vi "Lockin_time_data analysis.vi"(0 "File or Folder Path":path=path "G:/.shortcut-targets-by-id/0B8-gGFa6hkR4XzJJMDlqZXVKRk0/ansom/Data/PPMS 3/SA40511C.20250205/01-Rwire_BsweepTsweep", 5 "offset":i32, 7 "length":i32=1, 9 "index":T4={"I+(A)"="X2", "I-(A)"="X5", "V4T+"="X1", "V4T-"="X6", "Top gate "="AO3", "Bottom Gate"="AO4", "Local Gate"="AO6", "B/Time"="Time", "X axis"="Magnet", "Temp"="Temperature"}, 11 "stop":bool, 12 "File Type":T3=enum."TDMS", 13 "decimate files":i32=1) -> (6 "V_N vs B":cluster{dbl[], dbl[]}[](graph), 8 "Gvs B":cluster{dbl[], dbl[]}[](graph), 10 "Gates and B":T1={"Top gate"=-2.38250399563554e-06, "Bottom Gate"=0.0, "Local Gate"=0.0, "B"=3821664573.0419946, "X axis"=2.999917578125}, 14 "Comments":string="Device: \r  Device Name: SA40511C.20250205\r  Computer: PPMS3DAQ\r  User: Ranjani\r  Instrument: PPMS 3\r  Description: |\r    LAO/KTO 3wire Nernst\r\rExperiment: \r  Time: 2025-02-06T01:02:54\r  Description: |\r    T = 100mK to 2K, 100mK step\r    B= 3T to -3T, 30Oe/s 0.18T/min\r    \r    Wire 2\r    I+/- = 2/5  1mV@13Hz\r    V+/- = 1/26\r    Wire 1\r    I2+/- = 3/4 1mV@13Hz\r    Wire 3\r\rSweep: \r- Loop1: [OFF, 0.000000]\r- Loop2: [OFF, 0.000000]\r- Loop3: [OFF, 0.000000]\r- Loop4: [OFF, 0.000000]\r\rWiring: \r- Electrode 1: Lockin 1, V1+\r- Electrode 2: Lockin 2, I+\r- Electrode 3: Lockin 3, I2+\r- Electrode 4: Lockin 4, I2-\r- Electrode 5: Lockin 5, I-\r- Electrode 26: Lockin 6, V1-\r- Electrode 27: Lockin 7, I3+\r- Electrode 28: Lockin 8, I2-\r\rLockin: \r  AO: \r  - AO 1: amp = 0.000 mV, DC = 0.000 mV, f = 13.00 Hz, phi = 0.00°, Sine\r  - AO 2: amp = 1.000 mV, DC = 0.000 mV, f = 13.00 Hz, phi = 0.00°, Sine\r  - AO 3: amp = 1.000 mV, DC = 0.000 mV, f = 13.00 Hz, phi = 0.00°, Sine\r  - AO 4: amp = 0.000 mV, DC = 0.000 mV, f = 13.00 Hz, phi = 0.00°, Sine\r  - AO 5: amp = 0.000 mV, DC = 0.000 mV, f = 13.00 Hz, phi = 0.00°, Sine\r  - AO 6: amp = 0.000 mV, DC = 0.000 mV, f = 13.00 Hz, phi = 0.00°, Sine\r  - AO 7: amp = 0.000 mV, DC = 0.000 mV, f = 13.00 Hz, phi = 0.00°, Sine\r  - AO 8: amp = 1.000 mV, DC = 0.000 mV, f = 13.00 Hz, phi = 0.00°, Sine\r  REF: \r  - Lockin 1: f = 13.00 Hz, phi = 0.00°, TC = 0.03 s, order = 2 \r  - Lockin 2: f = 26.00 Hz, phi = 0.00°, TC = 0.03 s, order = 2 \r  Sampling: \r  - Fs: 13000.000000\r  - N: 1000\r")   [LabVIEW 2020]
uses:
  <userlib>/LevyLab/LV-Data/LV-Data/Typedefs/File Type--enum.ctl
  <userlib>/LevyLab/LV-Data/LV-Data/Typedefs/Dictionary--cluster.ctl
  <userlib>/LevyLab/Graph Utilities/graph_utilities.lvclass/graph_utilities.ctl
  <vilib>/Analysis/2dsp.llb/Decimate (single shot, DBL).vi
  <userlib>/LevyLab/XY Utilities/subVIs/Sort (multiple).vi
  <userlib>/LevyLab/XY Utilities/subVIs/Moving Average (multiple).vi
  <userlib>/LevyLab/XY Utilities/subVIs/Moving Average (single).vi
  <userlib>/LevyLab/XY Utilities/Private/X Units.vi
  <userlib>/LevyLab/XY Utilities/Private/X Array Range to Index.vi
  <userlib>/_OpenG.lib/array/array.llb/Sort Array__ogtk.vi
  <userlib>/_OpenG.lib/array/array.llb/Sort 1D Array (DBL)__ogtk.vi
  <userlib>/_OpenG.lib/array/array.llb/Reorder Array2__ogtk.vi
  <userlib>/_OpenG.lib/array/array.llb/Reorder 1D Array2 (DBL)__ogtk.vi
  <vilib>/ptbypt/Probability & Statistics.llb/Mean PtByPt.vi
  <vilib>/Utility/error.llb/Error Cluster From Error Code.vi
  <userlib>/LevyLab/Graph Utilities/graph_utilities.lvclass
  <userlib>/LevyLab/LV-Data/LV-Data/LV-Data.lvclass
  <userlib>/LevyLab/XY Utilities/xy_utilities.lvlib
  <vilib>/Analysis/NI_AALPro.lvlib
panel:
  in  "Invert the voltage?":bool
  in  "Vac source":dbl=0.004 format="%#_13g"
  in  "Interpolate [T]":bool=TRUE
  out "R4T":dbl[][](graph)=[[0.000424230667060951], [0.0004241627892310994], [0.0004239762829222014], [0.0004240776446695195], [0.00042395565052737844], [0.00042385658657262767], [0.00042403039598027124], [0.0004240810092048603], [0.00042406297404835934], [0.00042399080114371296], [0.00042410664694500125], [0.00042424294917358654], [0.00042405440721684275], [0.00042383408715513976], [0.0004239805268122013], [0.00042402415538763007], [0.00042380226047949293], [0.0004238603471561728], [0.00042402239398964866], [0.000423794117176646], [0.0004236304354503625], [0.00042346014948994973], [0.0004237444893171298], [0.0004239119982147603], [0.00042374132535446846], [0.0004232669431588462], [0.0004233535579852907], [0.0004237016911869473], [0.0004235278148944421], [0.0004233387046453984], [0.00042341988853845095], [0.0004235810190481912], [0.00042377393067379845], [0.0004236998484156858], [0.0004234411722325005], [0.00042336227434465836], [0.00042284230554959625], [0.00042269568089598836], [0.0004231178707180585], [0.00042300293790850733], [0.00042312887072011487], [0.0004229865181367974], [0.0004227968712337211], [0.00042306796937519845], [0.0004230734327560945], [0.0004226940576570362], [0.00042303187675997786], [0.0004231402237564772], [0.00042302330197007846], [0.0004227341266901518], [0.0004226609130282922], [0.00042279282169723804], [0.0004226887479513664], [0.0004226007143430205], [0.00042281751346768805], [0.00042220939256442215], [0.0004224310454723942], [0.000422886802720675], [0.00042288719243734714], [0.00042248687396520237], [0.00042230013969068596], [0.00042248701149523454], [0.00042252762174203244], [0.00042213462135096694], [0.0004220214211054761], [0.000421841940937384], [0.0004222420680608442], [0.0004219888727551959], [0.0004219676480101798], [0.0004219551472359875], [0.00042195634242418414], [0.0004219040997890422], [0.00042167336464231077], [0.00042247972140130015], [0.0004217734936972054], [0.00042208245331560993], [0.00042186133268121986], [0.0004216840024900676], [0.00042171697083547265], [0.00042178861205538964], [0.00042174635123378817], [0.00042172819708202264], [0.00042146123224400136], [0.00042104818631271876], [0.00042132452616542573], [0.00042156672188832273], [0.0004213936319084997], [0.00042110757406554775], [0.00042101582832057923], [0.000421126048513413], [0.0004212305111095027], [0.00042121321174319284], [0.0004210727847972899], [0.00042082925795275324], [0.0004205614122592464], [0.0004206832818138018], [0.000420672623409281], [0.00042046085467745673], [0.00042043370400579415], [0.00042064689351364767], [0.0004206859123358853], [0.0004205934255169018], [0.00042053893480939296], [0.0004204424428299226], [0.00042065161930425493], [0.0004205456388994443], [0.00042039717085107063], [0.0004203493257046196], [0.000420088570159928], [0.0004197794538457051], [0.00042007680941531485], [0.0004198713154711518], [0.00041957391008587576], [0.0004199500766845846], [0.00041970821913994385], [0.00041965394641512756], [0.00041945465124392824], [0.0004190695861565483], [0.0004189152757994222], [0.00041915150252475525], [0.00041883616773839643], [0.0004191943999910526], [0.0004189212355334126], [0.00041900942584169543], [0.0004185778775840564], [0.0004187374538311991], [0.00041899865722139364], [0.00041872486220338235], [0.0004186616533653799], [0.00041903033349288097], [0.00041827326130003785], [0.0004185896191123761], [0.00041792731365065], [0.0004183883835834742], [0.00041810264683005545], [0.0004180743195753931], [0.00041804382684701056], [0.00041759386573979947], [0.0004176624109572106], [0.0004180606783485715], [0.0004179427561280086], [0.0004175654283592434], [0.00041759140297762244], [0.0004175035398462255], [0.00041733643730809455], [0.0004173107668617529], [0.0004174851447006786], [0.00041733379099204545], [0.0004169440632617724], [0.0004167785870382156], [0.0004169452376170638], [0.00041698873953780006], [0.00041695731825598604], [0.0004168198698435353], [0.00041671381916733816], [0.00041658332646485075], [0.0004163205412953218], [0.00041630564727615017], [0.0004164986060327017], [0.0004164936166641299], [0.0004164022211122646], [0.00041605340850815834], [0.0004158206266273258], [0.00041560195723605624], [0.0004155263738664587], [0.00041579368533072535], [0.0004159158772866023], [0.00041558725042476456], [0.0004155658402594451], [0.0004156858044120287], [0.0004154434252531913], [0.0004152107139460031], [0.0004150944904526775], [0.00041495691551716757], [0.00041446620996558615], [0.0004146220979361046], [0.0004142377607273932], [0.00041444559467206343], [0.0004140876171560672], [0.00041406365094836395], [0.00041408490514907337], [0.000414259671091113], [0.0004139030425346164], [0.0004138904113998248], [0.00041355240750973795], [0.0004131619935822429], [0.0004133622557350194], [0.00041352842653432015], [0.0004132267655508752], [0.0004132740838617142], [0.0004131464521133263], [0.00041324772751134863], [0.0004125109728278841], [0.0004126125273050463], [0.0004128907650330233], [0.00041257978936212476], [0.00041288285104010524], [0.0004120442854661527], [0.0004121762959166953], [0.0004122026469805812], [0.0004120518437036138], [0.0004116936384655424], [0.00041150879247894677], [0.0004115069337463857], [0.00041148441988028835], [0.0004114515803829334], [0.0004113060652839863], [0.00041108581901707746], [0.0004110906462329125], [0.0004110752703801405], [0.00041075390031276523], [0.0004106517640540189], [0.000410399631148385], [0.0004106787540272022], [0.00041014686908993745], [0.000409997211227693], [0.0004099814288044587], [0.00040996075953669673], [0.0004098489275993161], [0.0004093034831015724], [0.00040926613959019816], [0.00040939423361016213], [0.0004090823545464051], [0.0004087797494786075], [0.0004090603285344171], [0.00040844990205408916], [0.0004083652920861278], [0.00040809586619167825], [0.000408278861552735], [0.0004081282367228271], [0.00040766819187970307], [0.000407486833487587], [0.0004078195117538214], [0.0004073809028703732], [0.00040741251690592904], [0.0004072828407728622], [0.00040691531006533424], [0.00040670282933438523], [0.00040648670922814335], [0.00040616671198854935], [0.00040607534141184437], [0.00040567991514284783], [0.0004061555100845717], [0.00040549717362588624], [0.00040555775777520534], [0.00040552116622386003], [0.00040513027861203835], [0.0004048911519333559], [0.00040481876500362754], [0.0004049005250038757], [0.0004044985906450438], [0.0004044851792730337], [0.0004039740619559113], [0.00040411507059179204], [0.00040379943401415067], [0.0004036352712094941], [0.0004033223458971997], [0.0004029685391153389], [0.0004026727361235646], [0.0004025738373273037], [0.00040277125215388583], [0.00040261462748985124], [0.00040248701162581905], [0.0004019122478168556], [0.00040183032413019197], [0.00040176761061710005], [0.0004014073837945468], [0.00040113398973144656], [0.000401156537326922], [0.0004009407129078838], [0.0004003598931733455], [0.00040016491517679014], [0.00039990292432806254], [0.00040002656071556425], [0.000399436080539296], [0.00039899838986452615], [0.00039912060656544445], [0.0003988630746367092], [0.0003986696693290012], [0.000398509641924198], [0.00039807456712268795], [0.00039778933180974386], [0.0003978325136548987], [0.0003977994514087603], [0.0003975573123797153], [0.0003971316612401363], [0.0003966861233101917], [0.00039651260103685366], [0.00039646652935005657], [0.00039625949562690463], [0.0003960129700666822], [0.00039569447421889254], [0.00039540843318506793], [0.00039521855798382627], [0.00039503654429677066], [0.00039474946034926745], [0.00039449883536015254], [0.0003934596900016189], [0.0003938348258829759], [0.00039330907507062886], [0.00039302663769440844], [0.000393031660343259], [0.000392785492193626], [0.000392306074520132], [0.00039197668147137135], [0.0003917571817112346], [0.00039144799573972733], [0.0003912833561971956], [0.0003909645758493901], [0.000390361954193348], [0.00039024141520183216], [0.0003899451246795503], [0.0003896138860494582], [0.0003892706158905659], [0.00038898601689086655], [0.00038863695145544566], [0.00038827809126682313], [0.00038828304845013226], [0.00038751394203900694], [0.0003874537345979429], [0.000387348179777241], [0.00038720272787068463], [0.00038656879778816225], [0.0003861268228654339], [0.00038578926184294163], [0.000385364899453384], [0.0003850866360283177], [0.0003848823915147919], [0.00038460341102141934], [0.0003841569880424961], [0.00038409807992470225], [0.0003834815479533935], [0.0003833885356809578], [0.00038318959120923275], [0.0003827280832871418], [0.000382287004682189], [0.00038186571626712396], [0.000381684322184493], [0.00038128464419751116], [0.0003806811146241439], [0.000380159214689599], [0.0003798215059924444], [0.00037975031327899724], [0.00037915287064583554], [0.0003787455568660593], [0.00037856239382861066], [0.0003782568807205582], [0.00037768427167309915], [0.0003775124979456841], [0.00037706508914289787], [0.0003765262119188912], [0.00037642126356395456], [0.0003759499939634604], [0.00037547045826117725], [0.0003749634004238384], [0.00037443224834813926], [0.0003743345084622313], [0.0003740123640542184], [0.0003734003978123629], [0.0003728638384673503], [0.0003725213666642626], [0.00037207365352599385], [0.00037207458986416534], [0.0003717206088276145], [0.0003710419680610729], [0.0003703784893869718], [0.00037025487023126377], [0.00036905795994318793], [0.00036929302610954105], [0.0003681865217775876], [0.00036838177741834377], [0.0003675135622656043], [0.00036706158874110243], [0.00036686338568076417], [0.0003662128467785237], [0.00036547004837859666], [0.00036540869939641525], [0.00036497128497439414], [0.0003645862056111999], [0.00036401908623622984], [0.0003634087093765291], [0.0003630615458814052], [0.0003627515105773954], [0.000362231707061841], [0.00036141307162458933], [0.0003611890431082454], [0.00036122097156634955], [0.0003603896964214785], [0.00035945318522324123], [0.0003591453758339982], [0.0003590343719652696], [0.00035852072480853364], [0.0003575418634387359], [0.0003571543923033553], [0.000356617978531131], [0.00035580828078117917], [0.00035526064441351965], [0.0003548779656671357], [0.00035439013600775475], [0.00035369554748218806], [0.0003530639657660217], [0.000352584560554065], [0.00035208862525122576], [0.0003514581215134454], [0.00035109216806437254], [0.0003502640330343151], [0.0003503815552577112], [0.00034953950486245767], [0.00034837801955748887], [0.0003484490489490972], [0.00034754017227262826], [0.00034693161198036203], [0.0003467333545370518], [0.0003453783036168856], [0.0003454707863694764], [0.000345077839997471], [0.00034457115124496713], [0.00034352895267482575], [0.00034299062362575146], [0.00034249033116514737], [0.00034166478888213023], [0.00034115774917752744], [0.0003406033549173651], [0.0003397188387195162], [0.00033929979684687683], [0.000338769059651745], [0.0003381433002590036], [0.00033740499737485726], [0.0003366382023469847], [0.00033597771016464356], [0.00033495937546459384], [0.0003343986896526359], [0.000334160897404128], [0.00033381406603788516], [0.0003329457406478669], [0.0003323156503030835], [0.00033153798754654803], [0.0003309851767377942], [0.0003299645363335848], [0.0003297219753357686], [0.0003287724628228224], [0.00032824278342590994], [0.00032744999870828914], [0.00032676882314358147], [0.00032614641092008933], [0.000325063509617802], [0.0003244186579784517], [0.00032392695423726797], [0.0003231652769268252], [0.00032219796287456885], [0.0003215631884860437], [0.0003211460330833196], [0.0003200351837545043], [0.0003194529182659099], [0.0003189605376024078], [0.00031796201694762617], [0.0003174814864418628], [0.0003166361599722241], [0.0003158530568086246], [0.00031518372989347375], [0.000314272920361374], [0.00031381660048494054], [0.00031323193060844574], [0.0003124091885568034], [0.00031135462201489485], [0.0003111028749818271], [0.0003101235021456214], [0.0003086592133504303], [0.0003082890411631986], [0.00030743436321143227], [0.0003066341668106728], [0.0003058164984149693], [0.000304314942928123], [0.0003044822365764169], [0.0003031739797733006], [0.00030205621871181963], [0.0003017916803263362], [0.0003001840099123891], [0.0002994934570730883], [0.000299119984993732], [0.00029853608022536207], [0.0002974789892693471], [0.00029634279547494525], [0.0002958775589855584], [0.0002950101530799046], [0.00029367055078161503], [0.0002932324391508975], [0.0002925132576674778], [0.0002912757032189704], [0.0002906834931969996], [0.0002894036100276825], [0.00028844787084611744], [0.0002874554323630716], [0.00028719106531622856], [0.0002865350873484346], [0.0002855258036055373], [0.0002848058200287221], [0.0002838722210765081], [0.00028297123367817335], [0.0002822301482934531], [0.00028130177191271097], [0.0002799972260451611], [0.00027966553805210614], [0.0002788086964184743], [0.000277160420488283], [0.0002769813491227371], [0.00027627672978082274], [0.0002753701279196827], [0.0002744673564361394], [0.0002734430480078402], [0.0002726618947560801], [0.00027190317924607283], [0.0002708640230896114], [0.00027006637100374467], [0.0002692514724238953], [0.00026814906313525074], [0.00026749699836120766], [0.00026664594688061665], [0.00026595576264880794], [0.00026527343309037753], [0.00026414540885805947], [0.000263433992507381], [0.0002618827281923289], [0.0002615201356483052], [0.0002608944508112101], [0.00025976249596917797], [0.00025923333717455855], [0.00025748400085064366], [0.00025672605698001346], [0.0002562198406706887], [0.00025577495354601635], [0.0002547350185538724], [0.00025314057073216287], [0.0002522408538143009], [0.00025151691503778325], [0.0002507430863265714], [0.00024977356338541027], [0.0002484790897771253], [0.0002478303243859414], [0.00024716602629690123], [0.0002465607707833769], [0.0002445933138383846], [0.000244168896763534], [0.00024312569690756086], [0.00024208643731961105], [0.00024129785399200937], [0.0002409965913358826], [0.00023952579956087493], [0.00023863674211351265], [0.00023796214251897428], [0.00023715769217793275], [0.00023593901598198562], [0.00023500757369404894], [0.0002339766960858069], [0.00023308338473998613], [0.00023227356627119158], [0.0002311008621998084], [0.00023021276031489555], [0.00022953930273102616], [0.00022873452943136924], [0.00022793077635354628], [0.00022670742126669732], [0.00022581095800516286], [0.0002250608704334104], [0.00022420111547653845], [0.00022317772021603841], [0.00022227387040019912], [0.00022135331505048576], [0.00022011782223851754], [0.00021931549712627798], [0.00021830688481195583], [0.00021688571186096503], [0.00021653794620749687], [0.0002155662482707712], [0.00021432172453559548], [0.00021313224538343538], [0.00021286040071258794], [0.00021099168052889832], [0.0002102583342152759], [0.0002093874573389767], [0.0002082429457566122], [0.0002072294811470816], [0.00020609494554979654], [0.000204620972640438], [0.00020395784728419742], [0.0002027850786007009], [0.00020158234557697086], [0.000200480022384824], [0.0001996538551644377], [0.00019867963796897528], [0.00019744138559303712], [0.00019650443441756967], [0.0001956670829458778], [0.0001942931149229835], [0.00019285677730090548], [0.00019174460917493203], [0.00019068625370383382], [0.0001898073359733395], [0.00018843340192143947], [0.0001869649584117287], [0.00018601093300083814], [0.00018490500608399016], [0.00018379734164132282], [0.0001827735400399447], [0.00018162017076823065], [0.00018029981157801633], [0.0001792444761967672], [0.0001783078557436908], [0.0001774229877720386], [0.0001762644472453768], [0.00017524379517966205], [0.00017423008035198688], [0.00017278111857095308], [0.0001716794211032669], [0.0001708075033514633], [0.00016928166042012012], [0.00016871067757524694], [0.00016775772882037345], [0.0001658855606752773], [0.00016456339621057913], [0.00016364505730686815], [0.00016236093026095286], [0.00016071273126401684], [0.00015925433474384086], [0.0001585754052571205], [0.00015771036864333266], [0.00015624422939498905], [0.0001547415326996638], [0.0001534532831513347], [0.00015250087147563804], [0.00015082918443493624], [0.00014980194615045548], [0.00014857223831417967], [0.00014722062318276198], [0.00014613531867194914], [0.00014423805279896912], [0.00014299822817294926], [0.00014108240745199717], [0.00014020485548647138], [0.00013896996949185118], [0.00013756275310695842], [0.0001362026196338391], [0.0001351212847557397], [0.0001334173011605224], [0.00013152589864280816], [0.00013057631898468717], [0.0001293282675427901], [0.00012793749088569362], [0.00012629632593984605], [0.00012468231588582586], [0.00012370726572128872], [0.0001226231622353656], [0.00012066030079622765], [0.00011931709806231169], [0.00011810213447875122], [0.00011686814025133169], [0.00011559612327410578], [0.00011440217037088983], [0.00011323377993772738], [0.00011155841452133518], [0.00010958389089617873], [0.00010840832608343727], [0.00010686600901916549], [0.00010548087440015973], [0.00010393231939255927], [0.00010242654909648006], [0.00010092498008330534], [9.975764236291937e-05], [9.78522894954398e-05], [9.675933321965506e-05], [9.542658276285901e-05], [9.417782089591605e-05], [9.286276958448489e-05], [9.135079150016967e-05], [8.996217167008856e-05], [8.849469961013168e-05], [8.705660288019142e-05], [8.627562158458351e-05], [8.488424433758368e-05], [8.373172032238617e-05], [8.188878549933955e-05], [8.084299587127756e-05], [7.959880455957557e-05], [7.815394054159889e-05], [7.694535337456393e-05], [7.583211286350537e-05], [7.54706670474579e-05], [7.422794045271236e-05], [7.332719323460862e-05], [7.198180452237042e-05], [7.160296329640439e-05], [6.999612646112883e-05], [6.871570017201501e-05], [6.825266343779638e-05], [6.741809424114905e-05], [6.627593674022957e-05], [6.534627832793692e-05], [6.382836886709758e-05], [6.213869089904026e-05], [6.160129369564693e-05], [6.080791081357675e-05], [5.965058456594791e-05], [5.861201103846546e-05], [5.741135665554683e-05], [5.601171094270476e-05], [5.483511443814798e-05], [5.3754837746655366e-05], [5.292918419847967e-05], [5.1450302463767015e-05], [5.0160484237607194e-05], [4.905903397627097e-05], [4.766329582802028e-05], [4.6694374105956646e-05], [4.5466425105702526e-05], [4.46027095218285e-05], [4.3260241405513176e-05], [4.285448232912136e-05], [4.166288758158848e-05], [4.113484988145149e-05], [3.993704487068794e-05], [3.8649775596779206e-05], [3.7658929247081454e-05], [3.717073518123489e-05], [3.597164503713075e-05], [3.5282231783890264e-05], [3.4309939360699035e-05], [3.3382100486617806e-05], [3.247343575227049e-05], [3.1049490271171724e-05], [3.0327452413728784e-05], [2.9633365074154364e-05], [2.8630517555459588e-05], [2.7821003252617973e-05], [2.726087844012784e-05], [2.643759137021278e-05], [2.5639114445985972e-05], [2.4623756242805693e-05], [2.3716787587869286e-05], [2.3146808247333968e-05], [2.2802573811615468e-05], [2.2259376836896833e-05], [2.1480282375968075e-05], [2.017877508738909e-05], [1.9496952498947267e-05], [1.881750866887652e-05], [1.7287926796796818e-05], [1.669488001616329e-05], [1.528365814136939e-05], [1.4485541409557787e-05], [1.3570586380708496e-05], [1.2808631862191794e-05], [1.2205366716199873e-05], [1.0994999527493e-05], [9.907119895046247e-06], [9.494118505512546e-06], [8.692668582576415e-06], [8.300410090159417e-06], [8.166581973528358e-06], [8.076818984865841e-06], [7.96145953163224e-06], [7.694631621959209e-06], [7.486141831060578e-06], [7.404797248384721e-06], [7.2142807240205665e-06], [7.258003805898742e-06], [6.7667250676157145e-06], [6.488350890693058e-06], [6.253280862779892e-06], [5.902926644461266e-06], [5.520110509862492e-06], [5.223020425482454e-06], [4.788199670255989e-06], [4.559210459603563e-06], [4.64894156241433e-06], [4.3738319902327695e-06], [4.36381219110776e-06], [3.634138026295857e-06], [3.365128330350591e-06], [3.795820050550465e-06], [3.58832112510691e-06], [3.4474538582150982e-06], [3.3543737194787584e-06], [3.002111962105642e-06], [2.602203310033045e-06], [2.599078437059716e-06], [2.5857659334619043e-06], [2.426301843170098e-06], [2.526276889275073e-06], [2.3746923549647344e-06], [2.2030706695720644e-06], [1.7089976511665323e-06], [1.6826859557028633e-06], [1.5197044138190835e-06], [1.4073188197739512e-06], [1.151877314672022e-06], [9.59322981006373e-07], [7.88779177173877e-07], [8.16706759451805e-07], [6.595564530721812e-07], [7.059052408414894e-07], [9.486790995580837e-07], [1.1621952558731871e-06], [1.1399026355617557e-06], [1.2239834162192177e-06], [1.239372245835736e-06], [1.0054692885454955e-06], [9.680297985770274e-07], [9.68015912207168e-07], [7.696428597866494e-07], [7.76719747080534e-07], [9.906488000256292e-07], [1.0816940362216466e-06], [9.510779241177977e-07], [7.698173202159706e-07], [8.017030502223652e-07], [6.847717917058129e-07], [7.393067319101267e-07], [7.973603742011444e-07], [8.764198626279046e-07], [8.099311932982451e-07], [6.333462702819153e-07], [5.119634504496795e-07], [5.874485984882843e-07], [6.789442259959498e-07], [6.241330067059724e-07], [5.481819242874455e-07], [4.270350978006336e-07], [4.873997120408079e-07], [6.161391301145316e-07], [3.951330615223315e-07], [4.2119416642330233e-07], [4.783443622761206e-07], [4.831689277255301e-07], [5.118889537056137e-07], [7.35724489050188e-07], [7.019145157381035e-07], [4.2313544265058996e-07], [4.799387724947165e-07], [6.365839035500268e-07], [5.842236769747904e-07], [4.793671667835134e-07], [5.9529761264043e-07], [6.80800282272372e-07], [5.626791632136349e-07], [4.027082444381794e-07], [4.096988882535464e-07], [2.4080424351293194e-07], [2.8572165429371504e-07], [5.683598295813946e-07], [2.0212331023043394e-07], [4.2366783249610906e-07], [3.849042545437706e-07], [3.9371284118968713e-07], [7.015721527104987e-07], [8.847009255316223e-07], [3.3828508964771214e-07], [8.407080186921653e-07], [7.865362886674064e-07], [4.604706183506133e-07], [4.996743303557389e-07], [3.9591495389754493e-07], [4.135110269210714e-07], [5.9068787541888e-07], [3.3340606665706695e-07], [5.948005677881927e-07], [4.770544577088404e-07], [6.768124126170029e-07], [6.437234969633249e-07], [8.502430996755945e-07], [5.729094144633987e-07], [2.9862123681957425e-07], [2.947639907915355e-07], [5.143039094906086e-07], [1.182343252848226e-06], [4.183127717714022e-07], [3.465129418353584e-07], [2.9577896279675033e-07], [3.90018216503661e-07], [6.767755896692462e-07], [3.852208405005297e-07], [6.544711521432357e-07], [7.138984086945376e-07], [5.950018304577847e-07], [6.594670821755201e-07], [6.821181667841666e-07], [5.679826686122814e-07], [2.611658634053658e-07], [1.1371963427891437e-06], [7.240163849838985e-07], [4.809020965709172e-07], [2.0042600365207e-07], [7.241760694818813e-07], [1.671659918152343e-07], [1.9155267349481118e-07], [6.371550614353073e-07], [7.9865675066446e-07], [8.891069149152412e-07], [9.400271144163188e-07], [9.142226270999283e-07], [7.706368226945615e-07], [2.1628177552525816e-07], [7.353176313864618e-07], [5.862949466246314e-07], [4.1654867040306635e-07], [5.793481115538854e-07], [8.539206858694867e-07], [3.7252791579939896e-07], [7.243170034889387e-07], [2.46116367675097e-07], [6.929438731797003e-07], [4.409865575473359e-07], [4.7430504765852804e-07], [4.4515914499968206e-07], [5.438261646135137e-07], [4.90960080240887e-07], [6.036676817830889e-07], [9.41727175746919e-07], [7.949615334387953e-07], [7.595497112287841e-07], [6.330597393232099e-07], [2.688123602911933e-07], [4.083022444433669e-07], [5.554752413856337e-07], [7.65715868686713e-07], [8.94144682260798e-07], [4.532204478928403e-07], [4.586927445932051e-07], [4.829473695896096e-07], [7.239583054177577e-07], [7.460571506126555e-07], [4.414842919947111e-07], [5.094139191592924e-07], [5.55350579767163e-07], [5.747022932720591e-07], [6.608773240571154e-07], [6.112720143359096e-07], [5.782729672500846e-07], [6.53379961831691e-07], [6.194351457450979e-07], [5.719377035283786e-07], [1.980873941731337e-07], [3.057559736839308e-07], [6.423827420611275e-07], [3.7201638365201624e-07], [3.9726387740914993e-07], [5.275822575466578e-07], [6.678704786914505e-07], [6.807302299673205e-07], [4.249422462650813e-07], [5.507438865366423e-07], [4.0536245822671636e-07], [3.9670679257375335e-07], [4.712838880619789e-07], [5.568285538882636e-07], [5.107072777641489e-07], [5.14131362835047e-07], [6.034363488875709e-07], [7.938049173773062e-07], [8.069710006696999e-07], [3.9513050512716876e-07], [2.4032779747808047e-07], [6.297809801277765e-07], [6.143298217794819e-07], [6.422891071000619e-07], [7.579231938900894e-07], [4.0751597085089307e-07], [5.075593401426301e-07], [5.345623141162618e-07], [7.686545483544158e-07], [6.744990537157891e-07], [6.890071720898888e-07], [4.586040831873333e-07], [5.734746453520762e-07], [5.655966510153189e-07], [5.705273897222288e-07], [6.917024007829463e-07], [5.470006788966108e-07], [7.174356763722703e-07], [9.205194823164183e-07], [7.543901957524686e-07], [6.299061699832852e-07], [8.391923453121581e-07], [7.698735150616842e-07], [8.372114275570576e-07], [8.587759632307552e-07], [6.575974550535537e-07], [8.381396817492836e-07], [1.059637914736776e-06], [9.163077625129625e-07], [7.106424747184517e-07], [8.513056331287615e-07], [9.238653264561855e-07], [8.008234433896023e-07], [8.746191679209059e-07], [7.776427701764064e-07], [9.67321482069493e-07], [8.410474029451524e-07], [8.15406285912752e-07], [9.553339344058176e-07], [1.3256272616054458e-06], [1.3909692559851619e-06], [1.9671388307438336e-06], [1.8275840098671987e-06], [1.8797864449128537e-06], [1.86717041858784e-06], [2.3530573488659703e-06], [2.2327624638364644e-06], [2.257747599999772e-06], [2.5649045741815523e-06], [3.0002573415617294e-06], [3.2127022553959887e-06], [2.844787105695722e-06], [2.9335652896601054e-06], [3.020306896802329e-06], [3.4845413798845672e-06], [3.4165930694190935e-06], [3.455761011629034e-06], [4.235275774545709e-06], [4.158489076672884e-06], [4.52568572955211e-06], [4.3513151295958744e-06], [4.378070677655292e-06], [4.797005002985187e-06], [5.029854589590737e-06], [5.0114968826786205e-06], [5.59355786424736e-06], [5.84036961679963e-06], [5.617852539252543e-06], [5.653507765928836e-06], [6.2062692790896985e-06], [6.511401865278022e-06], [6.806652972591187e-06], [6.695553346222389e-06], [6.95057069974521e-06], [7.1858499262691734e-06], [7.909763800534066e-06], [8.067644871180977e-06], [8.709758899736036e-06], [9.739029982286095e-06], [1.0693908787588217e-05], [1.1433839740728209e-05], [1.272302450064622e-05], [1.3215156125616807e-05], [1.4756170840676726e-05], [1.5406864293359305e-05], [1.6487974441853515e-05], [1.7167956691268483e-05], [1.786521526795659e-05], [1.8946644903982933e-05], [1.953677817328997e-05], [1.9936834449026658e-05], [2.0148564311373906e-05], [2.1085096241702588e-05], [2.182396584419943e-05], [2.2442570380587382e-05], [2.3495322528087958e-05], [2.4451168842017983e-05], [2.487920796698616e-05], [2.510701752763551e-05], [2.6041706563301482e-05], [2.692913921091009e-05], [2.7808479735092684e-05], [2.8765684783065227e-05], [3.0442743786319736e-05], [3.1547783197323796e-05], [3.208571530428628e-05], [3.3302486728018804e-05], [3.4291298836841246e-05], [3.519385562896357e-05], [3.6484312230158976e-05], [3.7336662072805525e-05], [3.810497548910189e-05], [3.9439159500508524e-05], [4.0797062771157246e-05], [4.158470109182966e-05], [4.218951989677827e-05], [4.3182031883051884e-05], [4.436554372531442e-05], [4.542041231937313e-05], [4.689111416146163e-05], [4.8073458777338275e-05], [4.915176709724156e-05], [5.040616699730321e-05], [5.1939243858192325e-05], [5.295651376471855e-05], [5.3837652850927716e-05], [5.4890355515985166e-05], [5.594301289539325e-05], [5.7128391024532475e-05], [5.8359429504993354e-05], [5.939567972514849e-05], [6.084058541037029e-05], [6.15114288322981e-05], [6.257896462962362e-05], [6.374021447607623e-05], [6.463625111861934e-05], [6.614068015427458e-05], [6.71776340361952e-05], [6.815801931591448e-05], [6.924163698488473e-05], [7.052469222248068e-05], [7.132572464734834e-05], [7.213040832263535e-05], [7.314307296747001e-05], [7.414910643765955e-05], [7.525145221524857e-05], [7.639575446310041e-05], [7.767765987925699e-05], [7.913565132351604e-05], [7.984959683044057e-05], [8.143257501721219e-05], [8.291521623968446e-05], [8.38793104833986e-05], [8.555518021713195e-05], [8.64741442872308e-05], [8.774808809805972e-05], [8.944758500778549e-05], [9.071140536789768e-05], [9.197431781411876e-05], [9.311360689409664e-05], [9.446897092959895e-05], [9.548180348224991e-05], [9.677261112290092e-05], [9.836106067789442e-05], [0.0001000400480382832], [0.00010135614906926947], [0.00010304970101650572], [0.00010491184879061619], [0.00010596963300153688], [0.00010738366914245225], [0.00010910695129805977], [0.00011074522981524077], [0.00011170511697582305], [0.00011314321681430106], [0.00011510782066177714], [0.00011673031026867234], [0.0001179027450343234], [0.00011934336271909837], [0.00012049547686459537], [0.00012191059898507485], [0.00012357063821633594], [0.00012468439764152546], [0.00012590815191295142], [0.00012733113197935006], [0.00012870606932140766], [0.00013051808028791755], [0.0001317832608633878], [0.00013299198886112203], [0.00013459279148855149], [0.00013654459069900672], [0.00013780104998324994], [0.00013930924608407386], [0.00014040538065707937], [0.00014151742572527843], [0.0001431252088128156], [0.00014430942980652074], [0.00014586753146104153], [0.0001473191811475136], [0.00014869031000040416], [0.00014957097055376612], [0.0001508445999347651], [0.00015224229211640368], [0.00015362384267951935], [0.00015495095769594197], [0.00015618094490903428], [0.00015769908139104996], [0.00015923574245418], [0.00016060391288455576], [0.00016184196734643277], [0.0001630226393810753], [0.00016380498588283563], [0.0001647530420114026], [0.0001661980335687498], [0.00016760907010363854], [0.0001690914192258236], [0.0001699324930700834], [0.0001711568356246252], [0.0001722457424610822], [0.0001733904462849532], [0.0001751375428293092], [0.00017599664854158042], [0.00017640664174398623], [0.00017761694119971128], [0.00017881719195617348], [0.00017982832341277146], [0.00018082812873657203], [0.0001821851574219616], [0.00018315802993987257], [0.00018447186154901653], [0.00018588317757923514], [0.00018658576809365505], [0.00018736368684151461], [0.00018870953547828008], [0.00019046974290636405], [0.00019144211438256093], [0.00019259311098396504], [0.00019382673673452627], [0.0001953506475506462], [0.00019631528076179965], [0.00019712814963449566], [0.00019826751677123536], [0.0001998993311037189], [0.00020119597810594773], [0.00020241786039330793], [0.0002029273946336081], [0.0002042053888288232], [0.0002050541166154176], [0.0002068208527739462], [0.00020774263339839655], [0.00020867664892360675], [0.00020929862726596772], [0.00021019275988965266], [0.00021123352812649898], [0.00021259597707244766], [0.0002134088852080701], [0.0002141251950452402], [0.00021531932194222725], [0.00021666292030044596], [0.0002175691015937411], [0.00021865216014670645], [0.00021933487371161205], [0.0002199677237297614], [0.0002211633070888008], [0.00022243931422982302], [0.00022327889446418885], [0.00022416585347264178], [0.00022551104370530206], [0.0002263309719911915], [0.00022722591953103276], [0.00022779054317406818], [0.00022879849980874008], [0.00022966280474808436], [0.00023144331312000826], [0.00023199807649419094], [0.00023263058149122122], [0.0002337327211850661], [0.00023471497515412768], [0.00023570744224709456], [0.00023663528931673345], [0.00023733171159786984], [0.00023854816940050303], [0.00023846360066958738], [0.00023961612767425106], [0.00024109627183934929], [0.00024249642267897218], [0.00024280030953277595], [0.00024405900345083264], [0.0002446758294515487], [0.00024571658067404925], [0.0002466425930441957], [0.00024778590037263836], [0.000248794967716386], [0.0002498474062828601], [0.000251064161105765], [0.0002516934070234019], [0.00025256694064322945], [0.00025369824094488417], [0.000254585996998516], [0.0002556609900441695], [0.00025632435680395747], [0.00025720111417719627], [0.0002578377646309328], [0.00025899776904615896], [0.00025957467886779997], [0.00026053585487917526], [0.00026169343923190293], [0.00026242910554550957], [0.0002633926034302904], [0.0002638860576050269], [0.0002649955313080385], [0.0002661398202656719], [0.0002667439957568939], [0.00026751393405607216], [0.00026854806227376337], [0.00026946026509310156], [0.0002700872402515192], [0.00027090639242319535], [0.00027197239767549913], [0.0002731791285702309], [0.0002738442494716074], [0.0002745983350986947], [0.00027531381136539047], [0.0002759624429739891], [0.00027628198382844234], [0.0002780836714844205], [0.00027860849837806805], [0.00027932503964806996], [0.0002807032353588279], [0.00028148742263892486], [0.0002820657004040444], [0.0002830529904124172], [0.0002841183251943005], [0.00028513057062293505], [0.0002859937918173113], [0.00028666010214155725], [0.00028696467939586494], [0.00028772495074415934], [0.00028861477393673704], [0.00028950231373865574], [0.00029074550400324796], [0.00029177200145252716], [0.0002923794043802383], [0.00029346017904013607], [0.0002942571582295447], [0.00029535135009111036], [0.0002962042430191629], [0.0002966543724998828], [0.0002974941261117767], [0.00029858697124426957], [0.0002991905381626827], [0.00030010892247314935], [0.000300695635403127], [0.00030134816675877855], [0.00030275076154311753], [0.0003029901201015567], [0.00030435541448217956], [0.00030524450724741235], [0.00030569538802097086], [0.0003069421115836009], [0.0003077711675465085], [0.0003084817100538353], [0.0003095307983312798], [0.000310645961015512], [0.000310920575186891], [0.00031118038287620707], [0.00031223288160470587], [0.0003129333516157657], [0.0003140746352681633], [0.0003151755607612244], [0.0003160381354020595], [0.0003168200758604429], [0.000317240870215574], [0.0003176149071608818], [0.00031825379506758073], [0.00031919174379324035], [0.0003198562693894436], [0.00032029701602771815], [0.0003214151572945333], [0.00032215559492953605], [0.00032245757559340704], [0.0003235070560710099], [0.00032383620319871955], [0.0003251681785549432], [0.000325650129498533], [0.00032673904075930196], [0.00032694218048324986], [0.00032813517457017306], [0.00032901549469387185], [0.00032888997670315316], [0.00032979977879280805], [0.0003307690156918712], [0.00033097120678864177], [0.0003318627929280954], [0.00033230946054047536], [0.0003334178782318692], [0.00033393580555793], [0.0003342674187042445], [0.0003351458469974853], [0.0003361462876437575], [0.00033656602208331955], [0.0003372369927493625], [0.00033768008429913135], [0.00033779224871786895], [0.0003386987767505733], [0.00033977368118238527], [0.0003402665115029132], [0.000340566551480079], [0.00034117140422791495], [0.0003418995312603942], [0.00034294265040283066], [0.00034294485231363745], [0.00034389563851188685], [0.0003445130984709129], [0.0003455605388796892], [0.0003460698940089466], [0.000346487436552921], [0.00034688749851165864], [0.000347887514397925], [0.0003481897316307096], [0.00034854817780595004], [0.00034953177247034587], [0.00034984437441744196], [0.0003499846307628487], [0.00035082192682687634], [0.00035159168727072286], [0.0003525428195909993], [0.00035282518387692673], [0.0003534008244414065], [0.0003538209360779247], [0.0003541806903784156], [0.00035502544464712627], [0.0003558547409074999], [0.00035618531099556276], [0.0003565805605532791], [0.0003574491033807393], [0.00035774007108493736], [0.00035813704009681564], [0.00035855322331900376], [0.00035932109171641366], [0.00035979470785987025], [0.00036023213603158524], [0.00036068242888695424], [0.00036131308709935766], [0.00036159219489182906], [0.0003622462134611279], [0.0003631084100942671], [0.0003630056724418117], [0.0003641559954241835], [0.0003641374967606656], [0.0003647784772253824], [0.00036484651513773466], [0.0003656303672707447], [0.00036623110261032617], [0.00036668323914171123], [0.0003669819820165285], [0.00036707816732467176], [0.00036763452111730256], [0.00036849238786384103], [0.00036880980220750577], [0.0003690831892260379], [0.00036975597782479226], [0.0003699202130252964], [0.000370613934348175], [0.0003713174279459789], [0.00037177093083906994], [0.00037203203561625566], [0.0003720419644318112], [0.00037271450112875623], [0.00037287147992027853], [0.0003736645539064242], [0.00037345442660316155], [0.0003743529713460968], [0.00037467262965348695], [0.00037507038124820317], [0.00037557582654617136], [0.0003761109232846978], [0.00037641649430531757], [0.0003768690897126329], [0.0003775045266898493], [0.00037759459877013523], [0.0003775951289572508], [0.00037824875277498316], [0.0003787599761790296], [0.0003794086020932231], [0.0003796843976564716], [0.0003799491479732016], [0.0003800694435692771], [0.0003805764648390209], [0.00038062501435119536], [0.000380955049244189], [0.00038183886327724094], [0.0003825329668217438], [0.0003822810462225301], [0.00038237327390737517], [0.00038282751203871067], [0.0003836689154869977], [0.00038389273970353935], [0.0003842593356114341], [0.0003845354570628439], [0.0003853208547055031], [0.0003848545131587719], [0.0003852038654273554], [0.00038532959546851094], [0.00038594335774407614], [0.0003865689413823728], [0.0003861811954862287], [0.00038740981620786054], [0.0003874330362757978], [0.0003878229438870357], [0.00038812630039149724], [0.0003879908140258945], [0.00038830809665998413], [0.00038858046349332377], [0.00038869422668565395], [0.0003891012500014505], [0.00038924522453701445], [0.00039021162234420125], [0.000390333190421396], [0.0003904955462819346], [0.00039088664688263373], [0.0003911149463710472], [0.0003909242825154873], [0.00039147048204058387], [0.0003921426200917066], [0.0003921859182454774], [0.00039255675709147937], [0.0003927624474867063], [0.0003930068951313384], [0.0003932834076364606], [0.00039386394036055634], [0.00039394884241666613], [0.0003940436542028144], [0.00039472982223055894], [0.0003949383623163986], [0.00039529699383178017], [0.00039547630322264206], [0.00039610761845424244], [0.0003961083668193948], [0.00039615116267917826], [0.0003965160085909853], [0.00039654497772288847], [0.0003969831833130594], [0.00039736022067575927], [0.0003973796204121996], [0.00039741469619916376], [0.0003978951350746367], [0.00039798210615752414], [0.00039832589191632735], [0.0003989638156194039], [0.0003991455004885013], [0.00039911093425236486], [0.0003992539067842909], [0.0003992060174534437], [0.00039988332922846954], [0.00040027387230313], [0.0004001089171355168], [0.00040054777844483676], [0.0004005837936820464], [0.0004008106117021775], [0.00040113282940083914], [0.0004013379371700021], [0.00040154354596498554], [0.00040157318820236576], [0.0004017775753475467], [0.00040194704035696326], [0.00040205032290030343], [0.00040221559149217814], [0.00040318864265971084], [0.0004027266419527885], [0.00040304644932861116], [0.00040318234987201285], [0.00040372077077823593], [0.00040366066881126025], [0.0004037557660843946], [0.000404123266981938], [0.0004042405490413119], [0.000404276215096844], [0.0004049214737983096], [0.0004054277690098495], [0.0004051746308349392], [0.00040541398994099005], [0.000405260179314013], [0.0004058126394047998], [0.00040568067983624926], [0.0004059061888114047], [0.0004061984152312922], [0.00040646063929292565], [0.0004064091560795026], [0.00040650466103296455], [0.00040636252781883417], [0.0004068448803501476], [0.0004068289187770198], [0.0004070494349279549], [0.00040724274317059076], [0.0004077189876041997], [0.000407728208304474], [0.0004081338704307671], [0.00040835139406007287], [0.000408277859799697], [0.00040840575667416677], [0.0004084512565993064], [0.0004089140537246629], [0.00040863971738826503], [0.00040897337945801495], [0.0004092324494347682], [0.000409189278172291], [0.00040889959598894483], [0.0004094737696533004], [0.00040946305091347], [0.00040973194813247063], [0.00040977616307570646], [0.0004102273187205077], [0.0004103116940414995], [0.00041039928731514914], [0.0004104541003031849], [0.0004101361450353799], [0.00041061283865515615], [0.0004109850889129508], [0.0004112470802473988], [0.00041134518986185695], [0.00041122186744771205], [0.0004115292659179654], [0.0004113891629621598], [0.0004114146730310007], [0.00041204488788107126], [0.0004121781502261846], [0.00041226124777975654], [0.00041252316762125567], [0.00041252893097986785], [0.00041225241913593955], [0.00041256918494793685], [0.0004124999072146794], [0.0004128919542243275], [0.00041287558705779576], [0.0004129840457542859], [0.0004128449692009831], [0.00041305318486734515], [0.0004128348104920292], [0.0004132128045103273], [0.00041385857198795827], [0.0004134364997377282], [0.00041377150404173815], [0.00041376377945456214], [0.0004135446080058277], [0.0004142294861485898], [0.0004140602208819621], [0.000414501920465728], [0.00041451062387576993], [0.00041488222819559354], [0.0004147439665612227], [0.0004149504236116926], [0.0004147151804973693], [0.0004150091119965207], [0.0004149053452293679], [0.00041524194268835127], [0.0004155844093778926], [0.00041525245169128053], [0.0004154565418193237], [0.0004154894710779567], [0.0004155811064412479], [0.0004156897929885518], [0.0004157018707187116], [0.00041574530783585574], [0.0004156959728131043], [0.0004161352141881701], [0.0004161988653942517], [0.00041598232651135844], [0.00041658078112172844], [0.00041622480013870294], [0.00041638769229320795], [0.0004165923902987015], [0.00041662079403947293], [0.0004163814154111907], [0.0004164523454185329], [0.00041693839788328914], [0.0004170352700772859], [0.0004170874234716866], [0.0004171338449904204], [0.0004171000627697213], [0.0004180118196104667], [0.0004176201670673793], [0.00041748809027059047], [0.0004173000287696173], [0.00041764038741116906], [0.00041770511246214446], [0.0004178937593197227], [0.00041820945979563565], [0.0004178477386291776], [0.0004182895278131472], [0.0004179422812040059], [0.0004180943519986947], [0.000418400528847837], [0.00041880847366003253], [0.0004187068360605128], [0.00041886359731105154], [0.0004189146598989344], [0.00041862896667195775], [0.0004189537239873918], [0.00041892354114387654], [0.0004194123929217217], [0.0004188059666226709], [0.00041904374891816416], [0.0004192007850383772], [0.000419368754925403], [0.00041960932507018864], [0.00041915314191687703], [0.0004195713860759216], [0.00041954674573615466], [0.00041975872595016137], [0.0004196553645087333], [0.00041942269365549824], [0.0004194705448619555], [0.00042008015447783767], [0.0004201181745318425], [0.0004202080879308917], [0.0004200616346280086], [0.000420061077536984], [0.0004204275823783604], [0.00042017131759302854], [0.00042074360751950135], [0.00042061843546958573], [0.00042057673084920416], [0.0004206464469614717], [0.00042089790142761093], [0.0004209704218554142], [0.0004208933645709644], [0.0004209189949460826], [0.00042085937761839124], [0.0004209512847778658], [0.00042094569665412966], [0.0004208749841165199], [0.0004213233212609629], [0.0004210498231095191], [0.0004214783167147095], [0.0004212573283792593], [0.0004212899887889277], [0.00042138819010773324], [0.00042123203395925577], [0.00042150620629219826], [0.00042133479360990754], [0.000421538693776576], [0.00042172478496850844], [0.00042162210279889377], [0.00042134728710882844], [0.00042141395728109113], [0.0004221331951188191], [0.00042225564266636334], [0.0004218928742075353], [0.0004213163377206349], [0.0004219252951130953], [0.00042195421288346676], [0.000422406173281114], [0.000422443524632059], [0.000422120285064228], [0.00042197272760086937], [0.00042201719405465354], [0.0004223963369015891], [0.00042259729037091094], [0.00042258443936732013], [0.0004226393720874725], [0.00042255063363991186], [0.00042247233088433134], [0.00042233156798118316], [0.0004222518223827484], [0.0004225224794478807], [0.0004228180624925305], [0.00042289125364881343], [0.00042310556601962186], [0.00042292611631186103], [0.0004225268646479593], [0.00042236389877858203], [0.00042254961636401607], [0.0004230890910058494], [0.0004231846553415174], [0.00042302309860566337], [0.000423101352031121], [0.0004234577728216894], [0.00042322439398164796], [0.0004231388375802842], [0.0004233238645386488], [0.00042326975134866665], [0.00042356554264091044], [0.0004235460601972066], [0.0004233028137891996], [0.0004229781489721747], [0.0004228847616283715], [0.0004232431307274036], [0.00042346527297686175], [0.00042358615048693145], [0.00042361612700710473], [0.0004237585300785523], [0.0004237510681135371], [0.00042305256136575606], [0.00042360685635638704], [0.00042322944897057324], [0.0004234455316459363], [0.00042350807301385376], [0.00042356247978676804], [0.0004236474811075484], [0.0004235030897810034], [0.00042343123267118114], [0.0004238032342910172], [0.00042396504192935327], [0.0004240508374919925], [0.0004239197409003764], [0.00042388292220658133], [0.00042379707188499113], [0.00042377986007313754], [0.0004242151093205872], [0.00042397528289167606], [0.0004241161388603782], [0.00042401715180025987], [0.0004241437369146205], [0.0004243907418808451], [0.0004244228571854587], [0.00042402436401608155], [0.0004244315605011509], [0.0004243214666556258], [0.0004245958948816251], [0.0004241302396020561], [0.00042428704810349517], [0.00042454973743908254], [0.00042432348511511344], [0.00042454646746346636], [0.00042430156305697846], [0.00042431626551169644], [0.0004244541083688822], [0.0004241714786307145], [0.00042499597855958276]]
  out "R2T vs T":cluster{dbl[], dbl[]}[](graph)
  in  "Averaging":dbl=1.0 format="%#_13g"
  out "R4T":cluster{"X-array":dbl[], "Y-array":dbl[]}[](graph)
  out "Nernst":dbl[][](graph)=[[131658.82678726746], [131680.75118340182], [131602.3490667736], [131621.16613217667], [131588.19421212125], [131536.7029603895], [131423.27915220393], [131307.19629681794], [131432.41914692693], [131398.61929603666], [131430.13501892437], [131631.7295429496], [131470.26024481462], [131438.2061474128], [131404.24394666], [131475.8133712486], [131522.74529861315], [131356.05572285585], [131345.30978580142], [131358.4853820989], [131359.42769200742], [131247.80381385074], [131375.23983074594], [131386.582709488], [131275.97881240584], [131117.17743233804], [131173.80964798704], [131224.31303561915], [131200.43187729776], [131088.5168103118], [131118.22534514958], [131186.43399649332], [131203.1317915321], [131211.0074281807], [131216.92571999072], [131097.57769110907], [130926.46247439782], [130968.97104759813], [131115.4769937623], [130907.54574069171], [131047.466531187], [131040.9833563629], [130911.3659360852], [130961.41993491635], [130981.00954512002], [130854.27458953054], [130908.24483239144], [130941.45704884599], [130974.84285060028], [130861.0465661708], [130755.95053338881], [130804.16824188194], [130897.38450674318], [130886.16011987209], [130774.91077455085], [130381.7253909792], [130525.58209508947], [130642.89204276158], [130875.19024964282], [130851.47766531885], [130712.88563184823], [130671.57309411615], [130760.84875412425], [130506.90539619581], [130347.94800248853], [130409.99832952711], [130475.95853381317], [130399.60381427148], [130458.57196635468], [130417.48471645798], [130298.2796076365], [130291.52491529078], [130161.11679538975], [130293.05277154161], [130349.68120102036], [130236.66760622038], [130219.09008172031], [130083.7967376909], [130120.68606341573], [130266.87124715868], [130255.74469222497], [130137.33172610345], [129960.00401003734], [129942.54005660758], [129916.82329976976], [130217.29755872823], [129884.22024625941], [129771.29761080294], [129819.93253485262], [129986.2120067], [130000.07587546088], [129865.99829485333], [129795.30811834926], [129762.6450385111], [129717.80649976249], [129800.63121265781], [129767.89937147638], [129594.8266175564], [129455.4765666947], [129486.19804540018], [129555.97993755546], [129589.3021957346], [129779.76399515332], [129464.87217874225], [129557.84743655892], [129540.79583587457], [129417.120709189], [129345.06498118662], [129267.40224498349], [129172.31906907677], [129386.13221656355], [129347.2652843635], [129278.62598334336], [129291.44843096961], [129060.52626758176], [128955.2022854649], [129047.07614481887], [128957.46975265688], [128819.91163235283], [128886.02159318728], [128928.78686586273], [128888.65843254264], [128827.49114185167], [128802.66789827675], [128675.2031605065], [128619.09909622527], [128636.91195100461], [128566.76805697246], [128538.84763535869], [128640.80767327762], [128394.91807328114], [128263.07890707254], [128215.93451526568], [128208.3315476569], [128258.11830380368], [128259.67586801633], [128200.91684620673], [128062.68337147277], [127999.81446395683], [128099.2349097642], [128120.24844893088], [128117.94021278864], [128012.72909247373], [127774.29005445803], [127740.76470137255], [127783.23960267959], [127754.73797244429], [127815.19819706227], [127786.19744935457], [127520.24896144528], [127464.20164527667], [127464.56424232866], [127516.13715141155], [127486.14218220398], [127462.15695223708], [127386.6974034641], [127180.47544122871], [127152.3409805963], [127188.01946176507], [127185.73943355898], [127207.71998721384], [127123.94604195622], [126994.01997441937], [126841.59953914874], [126715.06098940462], [126716.53445042302], [126753.86156915226], [126599.1882973478], [126571.0836827183], [126577.88429403483], [126525.99490617614], [126493.35440577079], [126440.0130095381], [126326.78846449472], [126252.67924273104], [126138.38457749637], [126120.9915083713], [126128.52445499037], [125964.12196843002], [125986.66841114676], [126007.09660280324], [126013.23060082617], [125950.71230950856], [125902.21323141422], [125641.51410931212], [125448.31659012802], [125523.94369343735], [125553.3926523279], [125424.96182986558], [125501.02145950428], [125420.08920109879], [125393.64562576084], [125045.91537471404], [125207.40173462394], [125084.89826781125], [124878.45686647085], [125080.74387330783], [124701.85232338095], [124708.81485087282], [124790.0899340193], [124712.30203480773], [124572.91539858379], [124528.39068601286], [124443.3617209852], [124340.49179809605], [124281.14482764495], [124265.65671590254], [124242.96918309164], [124171.32245077183], [124158.96257735812], [123966.17198543953], [123915.38630003862], [123873.24561739524], [123811.53887346968], [123610.72108699061], [123571.5278939008], [123461.0503339785], [123525.87299583826], [123283.58490309851], [123279.63717075266], [123238.083408468], [123107.30995104025], [122999.30636064187], [122930.86637101679], [122911.63309086602], [122769.99018353714], [122698.13508591449], [122554.97412067137], [122585.92386305414], [122501.61196650867], [122315.8483478746], [122239.11584070037], [122181.77337883651], [121951.65324090845], [122018.61064365112], [121887.87580512803], [121727.01249612101], [121661.33229159513], [121533.98459609339], [121354.673842797], [121383.00797613467], [121191.80310242032], [121274.92453331313], [121146.27336669168], [121123.89337360475], [120922.03115251094], [120808.5427428172], [120808.65700119834], [120809.53550279404], [120667.36047777093], [120406.18832483533], [120280.46716983951], [120249.58576998387], [120187.25050237731], [120025.4143233262], [119973.2358995062], [119872.8714993043], [119634.24278831283], [119400.86734829827], [119421.9080054388], [119421.40222463198], [119323.38518892883], [119131.91957549224], [118834.80711746939], [118948.62647559693], [118961.36112009146], [118732.50161289364], [118631.68636667424], [118628.24789421802], [118439.8099972853], [118252.8200795554], [118095.10612885689], [117918.24802419021], [118052.69239759361], [117759.12510129642], [117561.68430622663], [117474.64660830474], [117415.00091846763], [117356.19089838774], [117241.27052381616], [117119.3029453409], [116976.71862611477], [116799.43523680081], [116701.55360925796], [116643.53067751147], [116489.11357438941], [116323.46835714958], [116230.18816954066], [116026.97223236835], [115825.30271796387], [115907.13792064821], [115763.44952893372], [115605.57058216332], [115412.99287118895], [115210.98673347617], [115136.89460589652], [114926.2174855013], [114550.82036301198], [114741.84767970424], [114501.90411410091], [114230.85015376513], [114220.65559397421], [114083.38032703479], [113867.85830254194], [113674.9605490878], [113481.99014325507], [113366.77000175379], [113368.04133838591], [113146.3677374392], [112798.7558578116], [112747.45826616709], [112637.99182789633], [112440.5519059222], [112244.6807162589], [112089.380345472], [111892.58077986902], [111696.1463784629], [111663.14440416751], [111449.31491089938], [111258.71611125284], [111109.61750387472], [111079.47805751157], [110706.88753855861], [110565.33369833091], [110376.66151721207], [110310.28345539384], [110273.56467887975], [110046.50393299454], [109727.71531881731], [109546.40901085621], [109447.65185651935], [109210.55222552974], [109099.65238665114], [109044.78373136655], [108752.38013374928], [108615.40033225057], [108439.45548344059], [108223.81189970001], [107992.46657195875], [107739.82287677281], [107530.00068886334], [107369.51048486383], [107289.86318815874], [107041.0342877041], [106813.35698459973], [106735.60413600758], [106449.20053080874], [106210.83702562598], [106032.0445730563], [105799.80344629467], [105618.44791348919], [105502.9753910623], [105258.41928022682], [105014.75322662534], [104754.23448700114], [104546.96584189666], [104355.21496862479], [104202.47456818662], [103940.92381982924], [103634.24686018174], [103538.30421572106], [103332.22484857342], [103278.58011611117], [103056.18380804693], [102808.00409215617], [102442.53613454472], [102314.3425891408], [101980.43923135435], [101831.18372979175], [101549.01845600168], [101502.96526028929], [101130.24992541882], [100817.8830831703], [100668.48927194119], [100387.33806688164], [100114.5192229267], [99955.28703547051], [99783.29090154848], [99526.15427805527], [99098.9639695284], [98825.23909891922], [98749.4506934658], [98619.60804133689], [98363.4384175733], [97990.71191845405], [97802.56670319205], [97746.07445619661], [97389.96792171871], [97011.81874822095], [96780.30824759061], [96655.73150653832], [96410.53643448491], [96023.58873720765], [95838.7788845751], [95577.45719565712], [95186.16367205924], [94998.65738413733], [94733.46833596978], [94503.97988593919], [94251.48667615317], [93959.53415932982], [93652.70038479936], [93289.1845453073], [92982.9957197313], [92846.2087989781], [92599.05892780378], [92503.0858123288], [92174.36438709662], [91637.00482246114], [91605.3665876037], [91208.99621596147], [90990.85208969888], [90820.9475969323], [90265.24083982791], [90275.42483553177], [89949.75662842183], [89727.41477656292], [89291.54476335195], [88996.54543514097], [88705.68100819789], [88367.23158958489], [88166.39466433473], [87903.843259302], [87507.85153534338], [87270.41649197797], [87021.5013573038], [86722.73820493808], [86411.63948315002], [86027.16442406044], [85794.95813014972], [85434.02986005883], [85119.57656709927], [84889.14501876163], [84698.67083702833], [84392.44748455507], [84002.89333182003], [83633.86719898325], [83403.26059892234], [82943.85372185161], [82926.10872402773], [82439.07549306998], [82193.50027362289], [81754.12536694488], [81497.94256914972], [81177.33724658878], [80774.76919751438], [80539.94182940327], [80285.5994189838], [79938.20542829503], [79527.29839441815], [79194.7500445217], [78977.29898158196], [78545.67680121989], [78270.6999693727], [78076.35626998433], [77726.1841946527], [77343.98133130652], [77000.10757633872], [76677.20292728863], [76380.92560770603], [76021.08209443881], [75822.76997856924], [75580.77963710974], [75260.52952961011], [74859.90071551206], [74617.37917223584], [74242.81319509166], [73775.11613381498], [73483.41973760213], [73082.86517388068], [72648.42292314646], [72372.26642708642], [71819.43912630022], [71756.65023221604], [71267.73892685222], [70845.07563847024], [70747.50585197125], [70137.98592495185], [69781.60493856814], [69598.19886965909], [69369.52432525063], [68968.20704565325], [68509.01969953135], [68256.78992227123], [67912.28847618552], [67443.05197889432], [67223.30813754896], [66927.26844073717], [66448.6620626238], [66147.7514861098], [65724.74041402564], [65389.777480009434], [65013.11027746255], [64875.695258114014], [64531.19061920477], [64145.6718877401], [63829.835312438096], [63525.13672248779], [63162.05132431722], [62856.67520200212], [62600.12910076187], [62077.275114780896], [61901.3327747297], [61512.181139415115], [60977.97085971298], [60805.86736960368], [60594.67765292794], [60199.066148309954], [59848.308250141825], [59491.66967638359], [59178.35170069599], [58875.626145333306], [58500.50366545708], [58200.574076194505], [57875.87761966066], [57495.4301125058], [57220.1589025556], [56914.28356506271], [56680.0539764708], [56376.06499692541], [56004.73245376648], [55730.381867848], [55264.82821723361], [55058.90289610926], [54813.83711981621], [54400.30083356441], [54211.01038988667], [53624.08585558358], [53380.23482204217], [53170.53989178982], [52913.82702209951], [52606.41470142392], [52076.75492832753], [51771.34171498606], [51513.52108667949], [51241.064870024595], [50917.21025934496], [50483.83128098083], [50220.15739666944], [49980.086686586284], [49654.40935255179], [49189.66164541291], [48964.50786112017], [48698.4700309521], [48353.90564400889], [48010.71071040644], [47875.82085188741], [47470.56653035448], [47133.599560213814], [46915.976008478145], [46590.47501194204], [46211.49309220494], [45922.64494834246], [45580.47794215556], [45275.47606431218], [45025.52284679565], [44670.2228012739], [44404.017802891394], [44186.7524554102], [43903.127905057285], [43606.41558754022], [43284.83435308359], [43002.92550656737], [42753.755117023924], [42490.192575747504], [42181.29878943613], [41896.21871777103], [41614.22956555805], [41286.6218969346], [41040.75630020316], [40711.217715801264], [40334.45432385888], [40148.40531450848], [39879.92309433073], [39519.70869676792], [39199.766386312614], [39101.19385131087], [38623.22045111603], [38350.572499046786], [38099.94984305704], [37766.024663496646], [37513.66789815544], [37169.00153711198], [36809.52931365411], [36594.30901633547], [36271.338736931706], [35980.725709071725], [35675.60264622379], [35416.18506182883], [35150.484325786994], [34842.27888696759], [34570.899213461205], [34310.09451736497], [33993.24368497807], [33656.13860363717], [33357.85555527203], [33076.00043225441], [32819.46126093725], [32484.747297934606], [32138.603693281464], [31898.237269932462], [31646.160690748464], [31348.98715020087], [31068.705316821863], [30772.267173911943], [30459.712062362378], [30186.68426016989], [29962.111184343485], [29729.68911685796], [29445.85793825037], [29189.82968952587], [28935.787967453824], [28612.57132617358], [28359.27112850162], [28138.11334440061], [27794.40741135121], [27642.89608823538], [27390.81280416623], [26999.33995137527], [26689.773681463317], [26460.348728409732], [26179.888043487008], [25821.98376369791], [25506.152667965926], [25348.815941957022], [25130.87245388721], [24809.59001278238], [24501.873268387597], [24233.83111076847], [23993.5834952894], [23670.098102634416], [23450.504812612395], [23184.490675037378], [22908.120862729327], [22668.669053290385], [22265.793480911052], [22016.11589914776], [21645.87185651391], [21464.497901060025], [21207.173399867006], [20935.119184896186], [20667.473730040732], [20448.084793039012], [20123.418965704932], [19782.418299273162], [19589.90879402877], [19343.68578542185], [19073.44290764547], [18767.6948668049], [18473.503885803588], [18275.611058752762], [18050.292869706034], [17708.45444544835], [17466.787320432162], [17250.995359093344], [17010.55317458479], [16784.826349163814], [16568.786260131998], [16344.311643549374], [16049.631500925614], [15710.649504794636], [15503.904926404604], [15253.962062775394], [15002.45069599029], [14743.647423783566], [14490.385453954192], [14229.309657089272], [14023.002241739372], [13718.39291944946], [13534.78310719039], [13316.126123808586], [13113.505392510993], [12904.023055536245], [12658.588655761603], [12426.858327353526], [12194.348763496148], [11968.960970047972], [11824.999137255705], [11608.735449654081], [11429.71925080473], [11145.845411901959], [10979.299962608427], [10784.19734661092], [10567.575939878292], [10383.022499166416], [10198.549650173014], [10141.430783280859], [9950.47671409125], [9807.595758365567], [9607.838183407448], [9543.296121604304], [9307.557801737594], [9110.70223466756], [9034.695950137499], [8907.265631699625], [8737.462930074907], [8603.69583852442], [8386.786613978555], [8147.164047506424], [8063.452215216113], [7946.2865300192425], [7781.210280058715], [7632.6469906372], [7459.511824367209], [7261.546873332946], [7096.315278084546], [6948.0617311219285], [6831.54206430508], [6628.353112032075], [6450.458455161296], [6296.551465587085], [6104.727236295174], [5965.584568039325], [5800.46291917233], [5680.053778213568], [5495.529989887343], [5433.778947600009], [5277.334930072724], [5199.026424768602], [5043.834407438372], [4871.993305602306], [4736.631272556263], [4670.789403961045], [4508.2417484399875], [4419.260354478969], [4289.489154068626], [4164.80307205411], [4042.149706616852], [3857.7776607758233], [3760.5542275394246], [3666.8867341938294], [3537.1086389742372], [3432.0916937691113], [3358.3908438974704], [3250.3119781065484], [3144.135861127511], [3013.564950186172], [2896.727968737348], [2824.8102421463727], [2778.587348555377], [2706.838070323825], [2608.1459897587115], [2445.2093779708575], [2357.482213870672], [2271.891763023556], [2083.5180481410375], [2009.2777088763128], [1836.3397833241356], [1737.3964079998582], [1624.4471677090414], [1530.7715301386115], [1457.5504153111242], [1309.7107571140807], [1179.0120491090904], [1128.7088959067773], [1033.1264661067041], [985.1949305737755], [968.3302453796812], [957.7165337718677], [942.3554114847922], [910.0570339037091], [885.1526659388362], [874.712787019211], [852.1555671645315], [855.4624379720543], [797.1980878894085], [763.9072538584238], [735.7313590633903], [693.7096402115603], [647.9258190124197], [612.8093169491365], [561.4691692309424], [534.292719054527], [544.5600100655402], [512.0941851301172], [510.7430187771599], [424.93766774474517], [393.37309161080304], [443.6533447641847], [419.35188106831515], [402.74691812028374], [391.56421455277723], [350.2636501539213], [303.38182059908695], [302.88489645213826], [301.16953404101963], [282.4368004379444], [293.8944578193306], [276.1172530600896], [256.0494993467073], [198.52583100963085], [195.4083236582381], [176.38550402085272], [163.19276807136063], [133.49113527109353], [111.13101297958377], [91.3561677044826], [94.58345170570205], [76.31991820622271], [81.65708731955874], [109.79022484934464], [134.51134706972383], [131.8704366218986], [141.51214648696575], [143.25399592038497], [116.2216539139861], [111.90421064499947], [111.93107604447958], [88.96984783572785], [89.73283892685495], [114.44410233632439], [124.95820837867443], [109.86644749960888], [88.90590751544485], [92.59948699101732], [79.08247978060997], [85.37118371708648], [92.10791659387435], [101.19668696582904], [93.52706859662445], [73.11653904193578], [59.099305064053624], [67.83729925257393], [78.3995925144426], [72.06229806422553], [63.285276707394026], [49.29104552741093], [56.28375123658205], [71.06841991685509], [45.61659067926219], [48.60386618652469], [55.184121449315654], [55.70824308624695], [59.04249034393171], [84.86230989218056], [80.95203888565723], [48.794653626700956], [55.336452104420424], [73.41910107802057], [67.37274757625163], [55.27769564670932], [68.65113108193138], [78.49871364288325], [64.87474997506405], [46.41751927915568], [47.2364391318294], [27.768865648069266], [32.92573774215995], [65.51343751948946], [23.299957732089048], [48.80198099776038], [44.348657895489694], [45.38268145522255], [80.85596512255758], [101.9468391489362], [38.96036979915362], [96.87001077147387], [90.61999138538877], [53.0194878282726], [57.510717543516805], [45.607464764676706], [47.619946293429535], [68.00931514831662], [38.367860487350704], [68.45632452195291], [54.8706875240022], [77.80858477781116], [74.06183433913122], [97.79706010636937], [65.86586763818863], [34.31881835942485], [33.86501863076303], [59.073750590442074], [135.72550573531063], [48.0043361873907], [39.73755991778323], [33.922606430849015], [44.73140639921387], [77.55771382394974], [44.11755777756363], [74.8736972966446], [81.65104110579396], [67.96347568554201], [75.19805814405476], [77.6267580023084], [64.43574116260945], [29.48872112982314], [127.55684581717703], [80.43687938289311], [52.828490268750684], [21.689988536751457], [77.92459380490584], [17.821908007913947], [20.271023427815127], [67.00972361877984], [83.68581250476812], [93.20096371795601], [98.753794639555], [96.22609696220712], [81.23003224858583], [22.822778089818527], [77.76970662996997], [62.129060562617646], [44.20239789016503], [61.59317575137009], [90.94615770267649], [39.743816283963874], [77.48051809244569], [26.47731564371691], [74.60372416320071], [47.690896504443785], [51.5544242942158], [48.71985446522118], [59.93058344098824], [54.338130223501906], [67.46031360741425], [105.86338900862528], [89.7972643417357], [86.36114303146124], [72.1488377040232], [30.762790369346348], [46.829002023321095], [63.791381560429556], [88.05198098774622], [102.85402896490305], [52.157657383985516], [52.782054663893085], [55.59402465099183], [83.36378662376698], [85.9091498062904], [50.85223397454034], [58.69241534841371], [64.00392000894112], [66.26414491596486], [76.19091838063702], [70.47802718504386], [66.667871597857], [75.33290298095869], [71.42439725357325], [65.91057677501956], [22.853954395713153], [35.24673309970027], [74.06334604473575], [42.894223784157596], [45.806820134689374], [60.81824714395764], [76.98133584844382], [78.47470462347421], [49.01217257934483], [63.528131042423354], [46.75546376957793], [45.754044981741515], [54.36988459897909], [64.27482803147481], [58.95176366476606], [59.33426944119853], [69.62418742684542], [91.57897235736948], [93.13544602266953], [45.61083752060694], [27.716223987939753], [72.70039138522691], [70.9189433463275], [74.10914312638032], [87.45717277146137], [47.03454388946163], [58.632627349269654], [61.72112117450323], [88.76304079530729], [77.91468878225145], [79.50868949002415], [52.92988653454607], [66.1789026678309], [65.27828897658858], [65.87927896179387], [79.85382212286521], [63.14177975229876], [82.76383177146737], [106.29879087612045], [87.16069166231405], [72.78594301026354], [96.91840170620306], [88.91129655310826], [96.68242131223468], [99.18848829465952], [75.96863877983041], [96.84821853286422], [122.48062485749237], [105.8998523764289], [82.08929148474144], [98.3969149540761], [106.87586798044144], [92.57561460061869], [101.17013593510514], [89.90456530490971], [111.84978468466402], [97.2955117062769], [94.29029969753742], [110.62022140097442], [153.54683935260772], [161.22329759468545], [228.04750236356233], [212.01004862272686], [218.1879122879251], [217.00174736063857], [273.4053619017262], [259.5492258501886], [262.606240327058], [298.6940342619402], [349.38840921209487], [374.15423388985903], [331.38174991739544], [341.8221842946954], [352.07111170815335], [406.1007703022886], [398.81591365857895], [403.28717177538925], [494.3839890672438], [486.13589066539316], [529.8738860805901], [509.7896333830873], [513.1405999182654], [562.9445666986966], [590.7200092717118], [588.4200260926003], [657.8374502427966], [687.8370304965094], [661.7337838067235], [666.427720337274], [732.1089668267653], [768.0091582177137], [803.585795679179], [791.5490595393868], [822.2931009482392], [850.4760290007895], [937.1535881216809], [956.6132316666726], [1034.070789493855], [1157.9307401654069], [1273.5810322265945], [1363.06455711681], [1518.4624279981506], [1580.880592058381], [1768.0931601801121], [1850.0436928531728], [1984.24502223642], [2069.413978408017], [2156.9562498654495], [2290.062255416834], [2366.1698315700082], [2417.442508129924], [2444.947955748188], [2562.583709250073], [2655.593119691678], [2738.539869361933], [2870.4840502972233], [2992.4172544066423], [3049.0877472772418], [3083.625073267125], [3201.751542089304], [3316.181276370855], [3430.149501758711], [3557.777982244883], [3775.5077506253565], [3918.67458682069], [3993.202183348893], [4149.697706063779], [4281.09565643715], [4402.331276263504], [4570.989346347417], [4687.942955664084], [4790.939217846684], [4967.7525498006935], [5146.263063434338], [5253.210899136204], [5341.863742144267], [5477.445534039208], [5636.9842861010775], [5779.730851318392], [5978.1973908739255], [6143.037657783365], [6298.716887364025], [6474.942927480429], [6681.10339472243], [6822.27037965921], [6947.431732006517], [7095.947755742993], [7241.672879195039], [7405.688927319941], [7575.226309609567], [7729.290868678926], [7930.995341384147], [8031.980450225353], [8191.0128443439135], [8353.650191380455], [8489.427723718765], [8702.861952367444], [8852.151808535697], [9004.67721854739], [9166.977233950789], [9358.983443175986], [9483.833814923952], [9611.508468383156], [9769.971351478232], [9925.044524792984], [10093.589863274763], [10271.376543622568], [10464.825137181846], [10682.883864779], [10806.74953966512], [11057.71905837658], [11278.855218561092], [11435.192787322967], [11697.383223675404], [11846.945441652673], [12055.29329633535], [12316.49303996947], [12517.34056788786], [12720.082089497464], [12908.832640229139], [13132.468511003317], [13299.839981485286], [13515.560670652743], [13779.159070487929], [14056.37327760077], [14275.914118383433], [14553.037350061162], [14865.889899490021], [15048.07956502611], [15311.132444790484], [15596.361279357836], [15886.780614221381], [16056.339078969018], [16322.459375534192], [16651.9202944603], [16951.54788104238], [17153.005901012428], [17432.45940545654], [17652.04877330738], [17903.19415548822], [18200.034878884464], [18423.152274718497], [18657.48350772973], [18917.972931016302], [19173.32960451025], [19513.91139239708], [19767.803626482928], [20005.423095748312], [20313.28104378862], [20682.618268829774], [20927.03100011918], [21212.328312201393], [21448.05120199351], [21688.270514303444], [21999.39672325492], [22248.39915052969], [22568.578192803758], [22861.343153860285], [23148.469878586715], [23356.685540109178], [23630.56351571031], [23919.322212999312], [24203.992168603683], [24485.417512546013], [24752.557997337855], [25082.794427899673], [25425.793604646264], [25716.90922631053], [25996.35055154483], [26247.331285025433], [26451.310112237796], [26694.42788401905], [27008.853139982955], [27311.687234690526], [27627.943984155925], [27846.389434831297], [28111.278544041234], [28382.57145785316], [28687.193667998545], [29075.84424461807], [29292.396045520123], [29420.309880931683], [29692.373012282726], [30004.68342796277], [30262.077524788885], [30484.41663200379], [30821.70041609923], [31089.7865360171], [31413.711676069892], [31751.53270726872], [31958.213660067697], [32190.082580750888], [32514.83032408401], [32907.812770281744], [33158.503017163675], [33485.966061383995], [33755.059538959365], [34162.61623177059], [34394.188519503245], [34634.86859213122], [34952.14340466249], [35356.31550477543], [35707.65434607316], [35974.297522571615], [36173.13283504913], [36521.83524898497], [36802.72955642827], [37238.116077788385], [37496.47703307574], [37754.58960573145], [37963.17824725721], [38190.31888883396], [38473.724821100936], [38882.51770684318], [39142.65542788709], [39344.803275936036], [39691.39587349835], [40039.871454724984], [40367.08593271318], [40650.886648439235], [40871.822542590475], [41097.199673226656], [41455.67534946197], [41799.69759934077], [42075.52138544406], [42354.868410340074], [42730.7467891858], [43006.36564169569], [43246.456611196576], [43472.23060625182], [43775.01932539531], [44070.74473723937], [44563.876885686324], [44756.174727978825], [44977.139932763246], [45309.96952226779], [45676.54179061868], [45927.65392624805], [46229.14328053309], [46505.81815550756], [46880.32140777187], [46956.59597959516], [47321.26577865129], [47766.70868705652], [48160.60065263098], [48323.22637667249], [48723.05440634983], [48974.32456627696], [49287.62938032066], [49623.17518074165], [49943.61187447025], [50335.62901067298], [50732.24002520472], [51078.86659080588], [51318.440999021084], [51649.20169532328], [52033.47861464836], [52344.59667253515], [52713.703238042406], [52958.03984219309], [53248.60200988691], [53508.537092524304], [53883.3200715835], [54128.445215037136], [54472.05240002967], [54886.68442581865], [55171.11953577248], [55504.87008392648], [55767.01669843966], [56168.74527125545], [56589.51276621567], [56800.201613510326], [57050.7426287786], [57403.014564012425], [57741.85250039967], [58018.150443149956], [58356.62284613592], [58724.02761033243], [59130.24212002565], [59434.22994785232], [59728.52389677965], [60050.19320621883], [60317.88218904676], [60497.27509417453], [61110.790937866834], [61294.09136707546], [61588.33404522365], [62116.0158434921], [62412.075031847904], [62656.52265976225], [63045.89522296874], [63401.10408816414], [63805.989045334005], [64186.73463065637], [64503.881258277885], [64653.16682740568], [64921.64939606973], [65301.295512493714], [65645.52604298887], [66090.20250122131], [66488.3445076905], [66788.15442741475], [67218.69384268673], [67509.44792679315], [67866.41886193152], [68242.91683928279], [68444.18768632354], [68799.37392332556], [69182.57512878165], [69577.48344496402], [69841.03438327719], [70248.09652745236], [70504.2544738939], [70960.61296307803], [71152.78460162338], [71629.30191940018], [72033.2364424933], [72170.50498401216], [72694.14578029781], [73073.93817987981], [73406.91699956341], [73839.19092611413], [74246.68361172124], [74424.95163763249], [74594.89106773271], [75025.31234891359], [75264.69465532205], [75712.49955810534], [76155.80257323032], [76593.94319416682], [76909.16821057448], [77094.64527030873], [77376.90006903803], [77677.20985450098], [78002.58791594362], [78375.31642158005], [78615.64885289565], [79054.82647724425], [79366.19871039671], [79536.92803631748], [79934.5864117854], [80202.50988926881], [80714.31946849704], [80999.01670346383], [81348.59165522171], [81462.68050202876], [82029.34871459522], [82330.90082442036], [82457.40155831038], [82852.84268311335], [83221.51877392734], [83397.40761467197], [83723.64309283214], [83985.78512664333], [84407.71248638775], [84705.58404277936], [84947.34921230213], [85322.7741927233], [85719.25883562764], [85893.07156990436], [86199.08219215994], [86471.72552029323], [86632.58579181146], [87046.39032052756], [87466.86909250966], [87613.61665560385], [87788.21801026512], [88182.54345296934], [88526.53785433041], [88899.52212267205], [88984.69741324236], [89446.11078644788], [89702.17829160475], [90180.43700371495], [90505.77901225415], [90644.85353022748], [90842.40351285631], [91275.03892713219], [91487.77135931914], [91629.86620766205], [92032.18224527861], [92319.20936286468], [92508.46300124796], [92806.2425740792], [93173.84251383261], [93481.59137495107], [93775.69837812924], [93910.9069387704], [94357.52020240128], [94429.0313293484], [94747.90621976789], [95027.15193483418], [95222.78928406515], [95482.0595733165], [95897.21504107605], [96017.51056248629], [96273.92544532598], [96530.40555196858], [96840.19843233707], [97162.2736778991], [97360.68950825365], [97620.84853088867], [97815.5417917826], [97912.73509234535], [98235.25876910007], [98607.01628212379], [98766.25208206495], [99199.54978327936], [99163.51752559983], [99618.57710531045], [99729.97680401323], [100021.88764838227], [100209.09189231206], [100421.6728576783], [100725.84556896436], [100867.9808631318], [101122.13123699176], [101454.52012288495], [101643.81091212176], [101790.37781259647], [102130.45035634677], [102239.53584879995], [102526.45843916544], [102889.45562963774], [103151.65648739361], [103292.59137515281], [103248.44012270958], [103632.54319426262], [103829.78718974206], [104090.37909094438], [104146.74434731448], [104370.60467682869], [104744.2126678394], [104974.98918687955], [105145.2681185547], [105230.22056023616], [105548.42693794055], [105612.79826432602], [106002.5420452521], [106159.8026654455], [106217.78951005828], [106611.2129779705], [106848.19809749497], [106948.90243940042], [107155.47938870075], [107329.31679013952], [107422.61406660103], [107643.42319611098], [107792.92284927066], [107976.92227667113], [108248.69423852651], [108645.74976471195], [108578.77957368853], [108655.65946275044], [109036.72158407967], [109218.4043168244], [109505.04433997681], [109595.22582248868], [109748.51724592522], [109967.97847257378], [110012.00992051106], [110111.18915437593], [110463.60751022275], [110578.11421898409], [110833.03268932494], [110954.31705536412], [111281.20641496958], [111132.14092389036], [111399.10013123241], [111659.82821101257], [111733.91261793977], [111910.73733220858], [112050.02641508338], [112174.85608049875], [112227.44939519295], [112507.00220395299], [112803.94463129704], [112947.87931976489], [113029.2896118048], [113125.77865475867], [113398.18201210698], [113319.85518403974], [113442.72414083606], [113858.4457217538], [113895.21556776836], [114034.8836143806], [114176.31107455569], [114332.64876417533], [114378.72087713201], [114687.78985862776], [114840.55646402019], [115022.69286313101], [115138.97157254121], [115296.51651593388], [115419.46302726437], [115558.81130170978], [115907.98770064916], [115955.34877913489], [115998.9023854126], [116235.28025352788], [116210.35849198181], [116467.64387615133], [116580.90192343034], [116705.57106792531], [116780.00610127625], [116932.28164315365], [117000.58638885395], [117185.20628544947], [117221.40632741184], [117402.6519766959], [117517.74191678649], [117666.41215787016], [117794.60687396806], [118016.33697108527], [118215.09425085215], [118139.17777434285], [118271.27832691913], [118425.46594205017], [118541.74972155827], [118641.02361695562], [118826.23615006829], [118884.63222949849], [118847.89328606227], [118932.623363755], [119053.48062355118], [119256.58277416704], [119217.23006947244], [119497.5122488031], [119600.73380646063], [119745.2171697454], [119868.90329957705], [120114.48761221576], [120131.08412282603], [120156.38694043132], [120254.0291097567], [120383.1398063602], [120505.95971773264], [120733.51741295189], [120820.50489044514], [120729.18277634405], [120851.89017027184], [120922.05037395192], [121238.98679153762], [121235.70805679048], [121249.75071196523], [121348.46235791603], [121522.68527233248], [121623.26932794481], [121707.28350485826], [121829.89225186272], [121897.61020327438], [121834.08811281883], [122017.04672538114], [121961.91023682669], [122275.25026061822], [122346.4103899739], [122400.51965127671], [122641.47245617026], [122632.35159953493], [122784.84758408093], [122746.95856855395], [123055.87342749319], [122863.30421505011], [122907.94199437175], [123104.92099672514], [123088.49317757392], [123047.5245673659], [123259.14234344309], [123231.99864473486], [123573.53843168932], [123440.80448356428], [123577.67609398397], [123674.0261673359], [123821.05298699134], [123819.20643386296], [123707.88456372137], [124048.48437646845], [124103.09974911797], [124060.82439571364], [124431.5666256426], [124330.25218749746], [124376.71121636979], [124545.00572571377], [124536.86116534253], [124617.11765136143], [124671.93219083836], [124857.59761109119], [124905.6058523477], [124925.11720363378], [124762.28144737604], [125088.13405732275], [125157.95368976983], [125192.06841225941], [125232.1795522994], [125319.63101106556], [125390.26975891234], [125489.7388198698], [125191.00208631092], [125377.31611540787], [125612.1407291419], [125524.30974323269], [125845.71243369757], [125747.18463657585], [125741.49569766728], [125981.04401200789], [126027.91594699692], [126236.33604254236], [126112.41625412149], [126136.30741467379], [126280.96164009057], [126419.83938301167], [126312.26702716433], [126313.5377757532], [126435.62651476629], [126567.36985492277], [126572.12257979813], [126665.66735561889], [126873.8574312323], [126764.29186067429], [126802.94968766392], [126747.51357839725], [126788.57717950318], [126918.47991749426], [126973.71249540853], [127179.71961336964], [127148.38780161821], [127091.65127181026], [127397.86442222571], [127286.3405028074], [127393.20210119578], [127274.0330725595], [127319.31537465069], [127398.38714535962], [127491.55192101185], [127499.2641721584], [127610.0393311385], [127693.93284265867], [127652.20299976147], [127650.50581339607], [128013.10606664194], [127974.44520270824], [127858.31642726215], [127885.84674831478], [128000.72886417941], [128129.53913261059], [128166.60730759447], [128277.03436494335], [128278.50722549984], [128264.41435465215], [128299.08778500668], [128333.97966819172], [128497.65614942902], [128523.8308523847], [128521.16617688492], [128584.51639119931], [128684.39777110232], [128615.6367248453], [128675.53795268992], [128729.78676199765], [128938.75925072095], [128694.32006390151], [128753.14698350357], [128739.11354800506], [128937.0305512456], [128928.48832479102], [128993.49090992553], [128878.36793372795], [129212.6466113669], [129168.74170500929], [129144.9762337708], [129049.98787907512], [129152.55625475396], [129345.21721613548], [129391.52819677629], [129470.28513291005], [129367.87627733128], [129299.73599298552], [129465.65354991019], [129549.00065713646], [129737.9615074435], [129723.94103762516], [129757.82836598481], [129465.20949131584], [129594.12171820132], [129753.72931487595], [129802.44458043734], [129802.63376696424], [129821.65990603826], [129744.27638305601], [129883.14574579931], [129875.0863891151], [129823.67922206385], [129811.28860416809], [129958.14006335127], [129940.74289817605], [130020.389247619], [130065.12806770737], [129976.63179359947], [130029.77239817797], [130106.78100710938], [130204.86719609088], [130221.25573040308], [130128.27279103678], [130183.6549061784], [130164.32050231422], [130407.74464319741], [130293.33706932804], [130238.73377647417], [130261.77394375768], [130457.89716211417], [130332.47417825118], [130510.97716077331], [130590.22433252075], [130420.42751868462], [130316.67956005911], [130495.03740683621], [130641.62861014994], [130531.7022256256], [130621.83041468498], [130820.69521410187], [130737.70698801083], [130679.08929117517], [130628.42996300822], [130548.62675666428], [130708.70628621173], [130720.58479749123], [130741.27692132641], [131026.17298586904], [130786.05918506767], [130752.23327731524], [130684.4858739622], [130647.87961127984], [130799.98589898166], [131020.48306031483], [131012.6675066644], [130965.37598745637], [131026.26255856779], [131074.76678407658], [131103.24312856665], [130948.41546636265], [130968.79914010272], [131056.16946379872], [131026.7539367774], [131042.89778547673], [131009.00412240223], [130908.26687155872], [131189.01183180156], [131181.94029407532], [131199.6923124649], [131320.0037783002], [131132.99891882035], [131305.9462640428], [131061.23915827568], [131295.27338418688], [131050.85920011836], [131177.52632851506], [131259.2698550421], [131359.67847954598], [131272.2703663133], [131194.59544073266], [131338.28257442158], [131402.59439298994], [131475.85245868273], [131513.0504014756], [131407.22437195433], [131403.2014030782], [131460.70731181902], [131360.0783231405], [131414.30176921538], [131493.10195949321], [131434.75777751778], [131485.18573547015], [131600.7472043373], [131652.35475715305], [131563.18916477257], [131473.39824188332], [131679.98524906728], [131972.067023933], [131771.41718274483], [131727.34062999574], [131687.40750133112], [131739.917844064], [131681.86239800404], [131834.42286680173], [131827.0670472562], [131838.10684582824], [131771.73862077747], [131798.05897154997], [131809.43016957364]]
  out "V/I vs Vsg":cluster{dbl[], dbl[]}[](graph)
  out "R vs 1/B 2":cluster{"X-array":dbl[], "Y-array":dbl[]}(graph)
  out "Waveform Graph 2":cluster{"f0":dbl, "df":dbl, "magnitude":dbl[]}(graph)
  out "R vs 1/B":cluster{dbl[], dbl[]}[](graph)
  out "R vs B out":cluster{dbl[], dbl[]}[](graph)
  out "Diff":cluster{dbl[], dbl[]}[](graph)
  out "Sum":cluster{dbl[], dbl[]}[](graph)
  out "R vs Bsym":cluster{dbl[], dbl[]}[](graph)
  out "R vs B Anti":cluster{dbl[], dbl[]}[](graph)
  out "I V4":cluster{dbl[], dbl[]}[](graph)
  in  "decimating factor":i32=1
  out "I vs  B":cluster{dbl[], dbl[]}[](graph)
  out "Temp vs Field/Time":cluster{dbl[], dbl[]}(graph)
  in  "length":i32=2000
  in  "index":i32
  out "Data (Dictionary)":T2[](array[typedef])=[{"key"="Time", "value"=variant(dbl[] array[1789 elements])}, {"key"="Temperature", "value"=variant(dbl[] array[1789 elements])}, {"key"="Magnet", "value"=variant(dbl[] array[1789 elements])}, {"key"="AO1", "value"=variant(dbl[] array[1789 elements])}, {"key"="AO2", "value"=variant(dbl[] array[1789 elements])}, {"key"="AO3", "value"=variant(dbl[] array[1789 elements])}, {"key"="AO4", "value"=variant(dbl[] array[1789 elements])}, {"key"="AO5", "value"=variant(dbl[] array[1789 elements])}, {"key"="AO6", "value"=variant(dbl[] array[1789 elements])}, {"key"="AO7", "value"=variant(dbl[] array[1789 elements])}, {"key"="AO8", "value"=variant(dbl[] array[1789 elements])}, {"key"="AI1", "value"=variant(dbl[] array[1789 elements])}, {"key"="AI2", "value"=variant(dbl[] array[1789 elements])}, {"key"="AI3", "value"=variant(dbl[] array[1789 elements])}, {"key"="AI4", "value"=variant(dbl[] array[1789 elements])}, {"key"="AI5", "value"=variant(dbl[] array[1789 elements])}, {"key"="AI6", "value"=variant(dbl[] array[1789 elements])}, {"key"="AI7", "value"=variant(dbl[] array[1789 elements])}, {"key"="AI8", "value"=variant(dbl[] array[1789 elements])}, {"key"="X1", "value"=variant(dbl[] array[1789 elements])}, {"key"="X2", "value"=variant(dbl[] array[1789 elements])}, {"key"="X3", "value"=variant(dbl[] array[1789 elements])}, {"key"="X4", "value"=variant(dbl[] array[1789 elements])}, {"key"="X5", "value"=variant(dbl[] array[1789 elements])}, {"key"="X6", "value"=variant(dbl[] array[1789 elements])}, {"key"="X7", "value"=variant(dbl[] array[1789 elements])}, {"key"="X8", "value"=variant(dbl[] array[1789 elements])}, {"key"="Y1", "value"=variant(dbl[] array[1789 elements])}, {"key"="Y2", "value"=variant(dbl[] array[1789 elements])}, {"key"="Y3", "value"=variant(dbl[] array[1789 elements])}, {"key"="Y4", "value"=variant(dbl[] array[1789 elements])}, {"key"="Y5", "value"=variant(dbl[] array[1789 elements])}, {"key"="Y6", "value"=variant(dbl[] array[1789 elements])}, {"key"="Y7", "value"=variant(dbl[] array[1789 elements])}, {"key"="Y8", "value"=variant(dbl[] array[1789 elements])}]
  in  "SE?":bool=TRUE
  out "Path":path=path "G:/.shortcut-targets-by-id/0B8-gGFa6hkR4XzJJMDlqZXVKRk0/ansom/Data/PPMS 3/SA40511C.20250205/01-Rwire_BsweepTsweep/SA40511C.20250205.000000.tdms"
  out "counter":i32
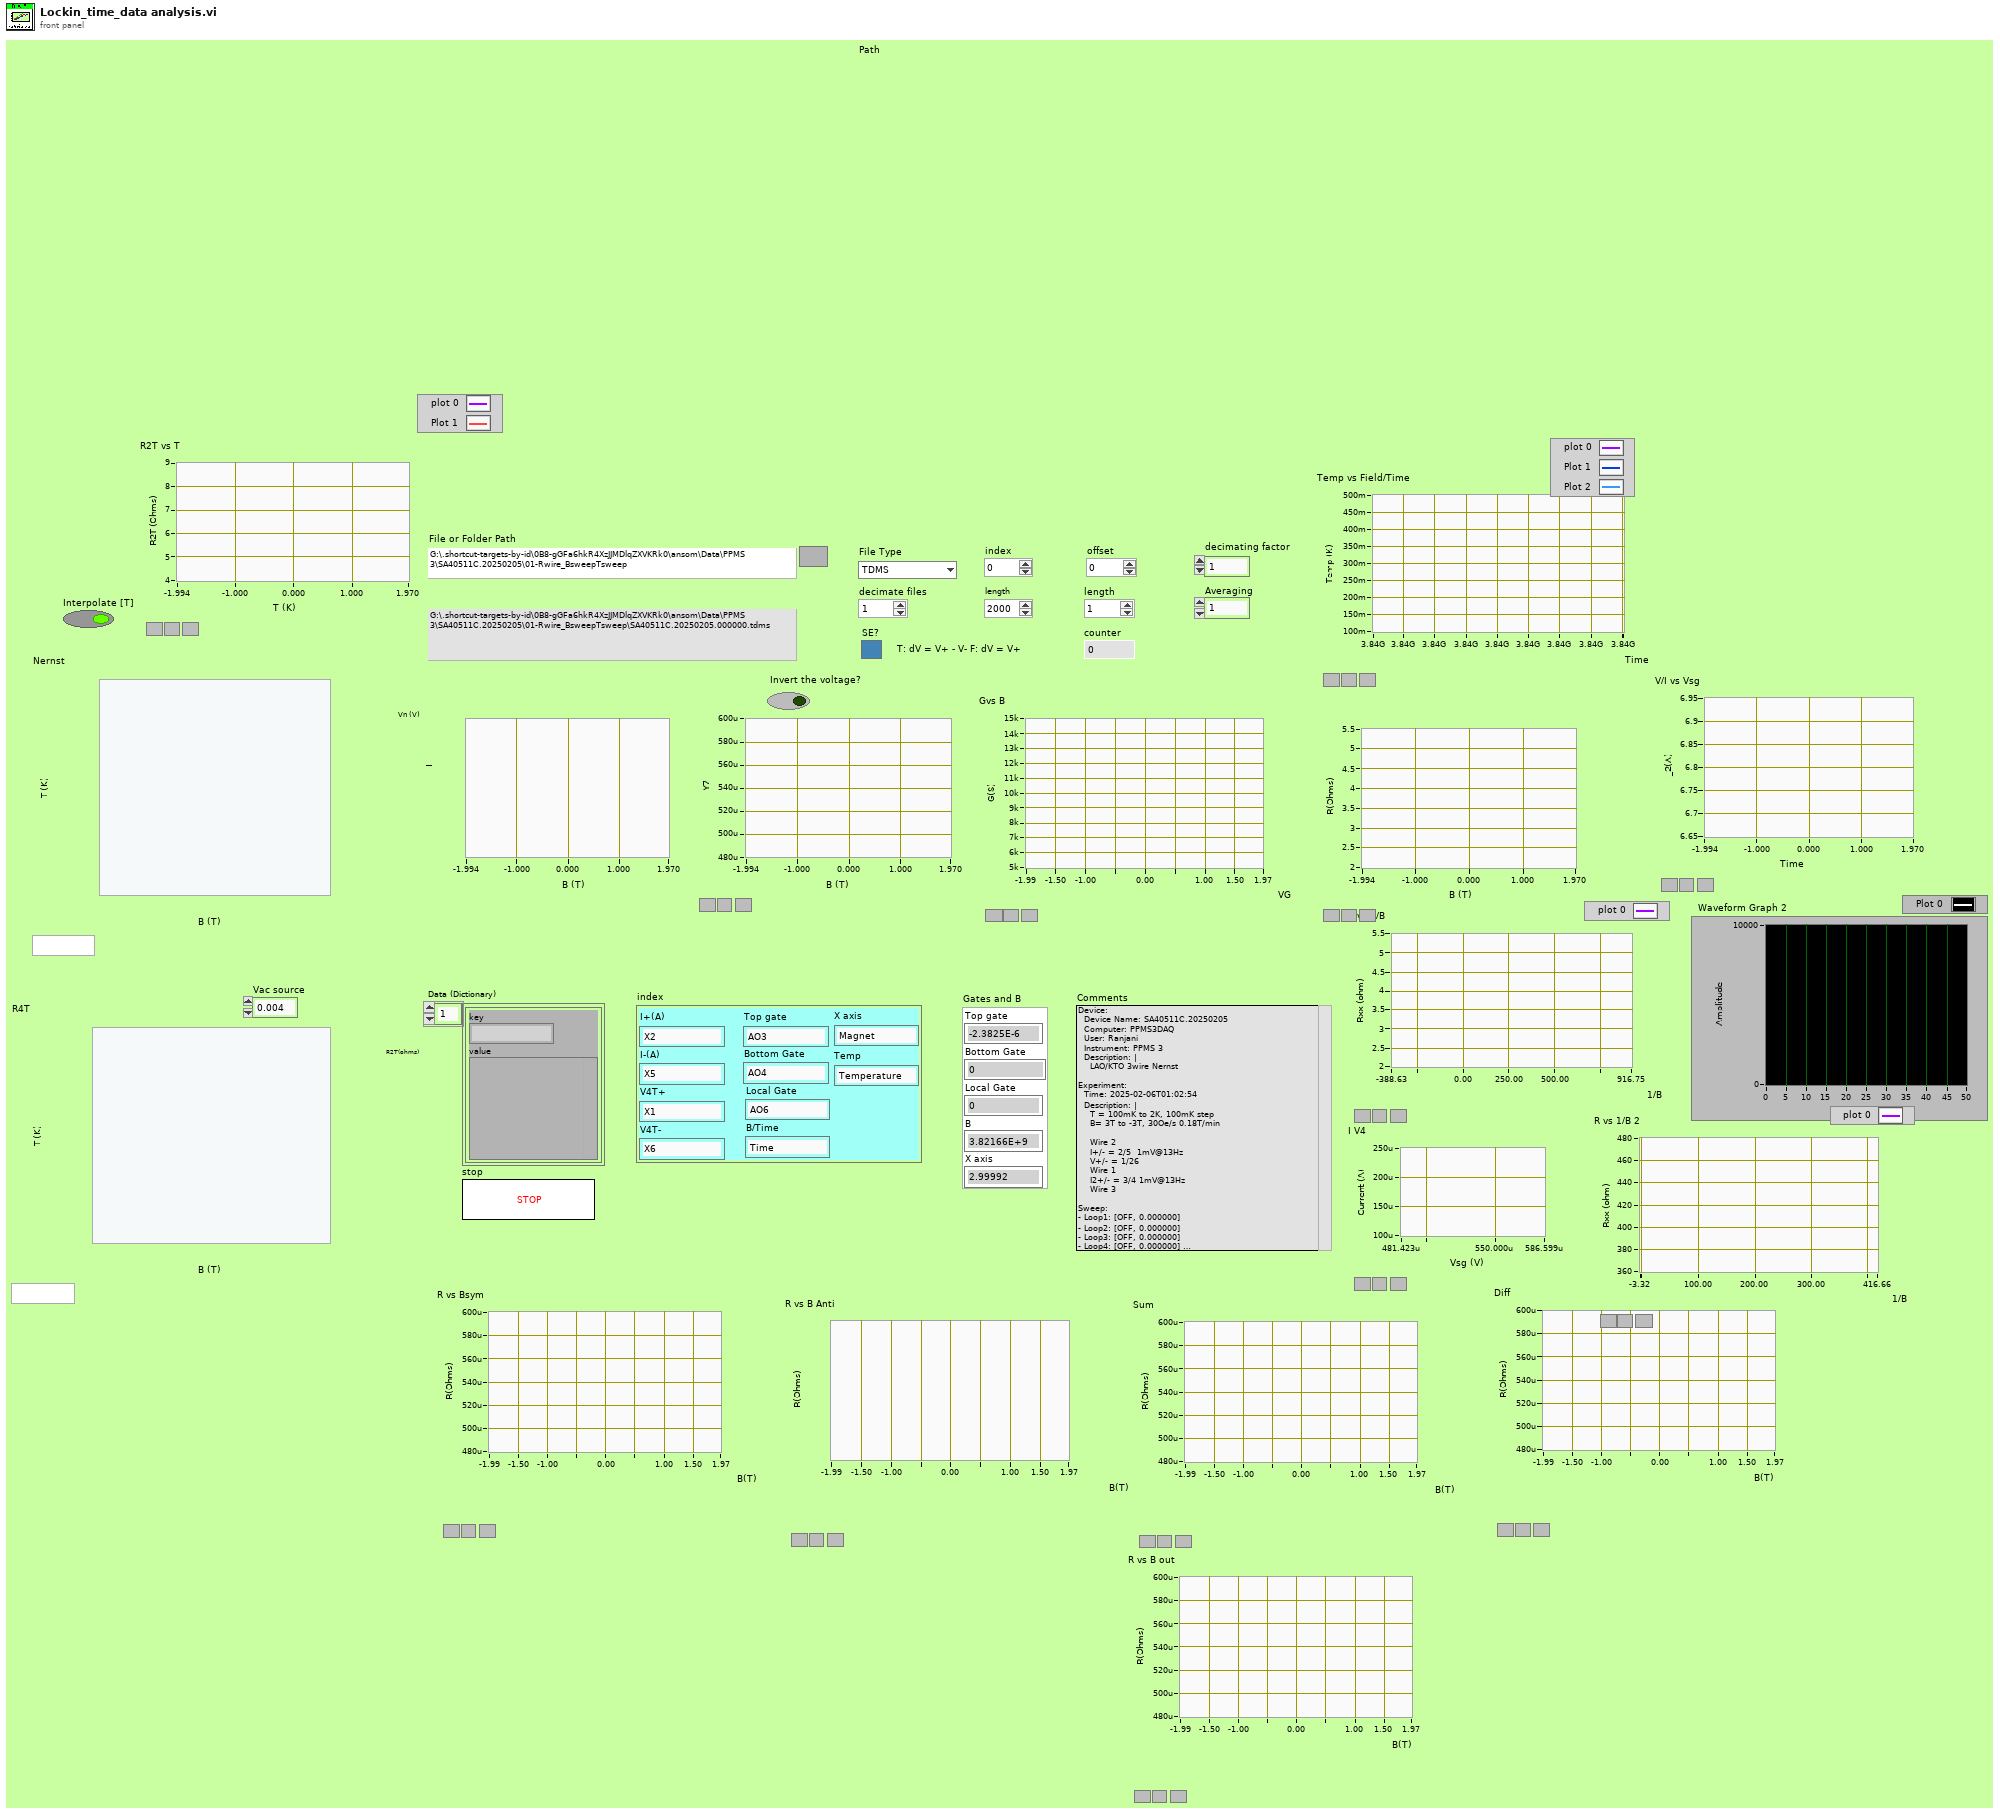
[diagram p1: front panel]
types:
  T1 = cluster{"Top gate":dbl, "Bottom Gate":dbl, "Local Gate":dbl, "B":dbl, "X axis":dbl}
  T2 = typedef "LV-Data.lvclass/Dictionary--cluster.ctl" = cluster{"key":string, "value":variant}
  T3 = typedef "LV-Data.lvclass/File Type--enum.ctl" = enum16{"DAT", "ITX", "TDMS", "VI"}
  T4 = cluster{"I+(A)":string, "I-(A)":string, "V4T+":string, "V4T-":string, "Top gate ":string, "Bottom Gate":string, "Local Gate":string, "B/Time":string, "X axis":string, "Temp":string}
  T5 = typedef "Dictionary Object RefNum__ogtk.ctl" = refnum<k1>
  T6 = cluster{"Decimated Array":dbl[], "Decimated Array":dbl[]}
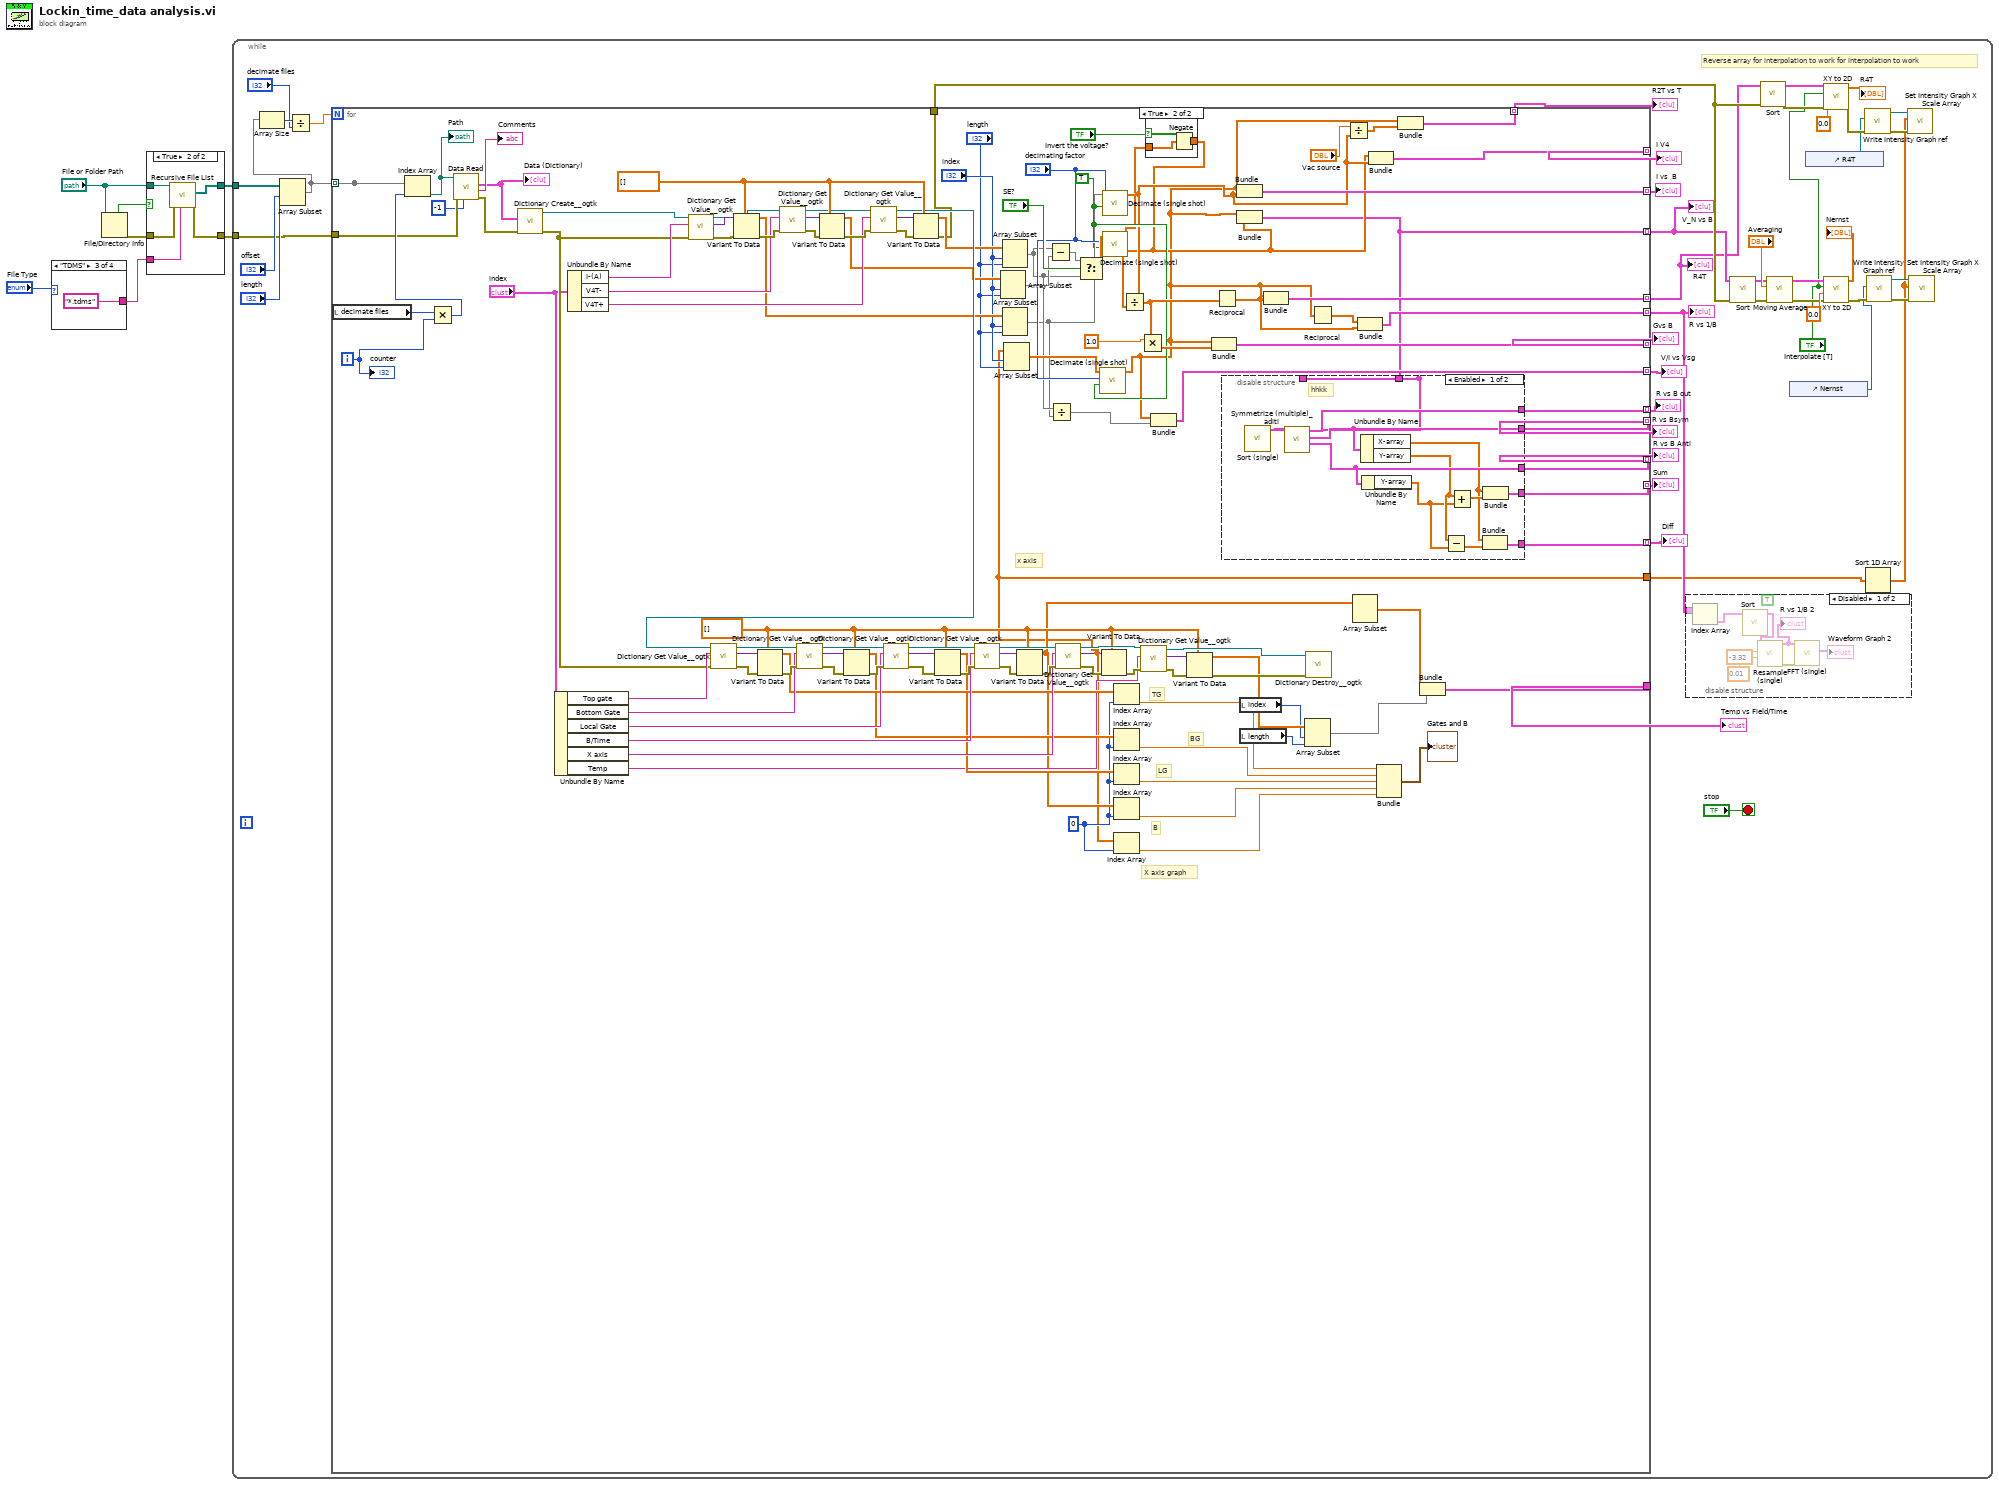
[diagram p0: block diagram]
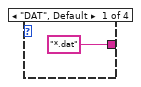
[diagram p2: hidden frame]
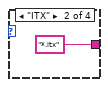
[diagram p3: hidden frame]
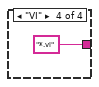
[diagram p4: hidden frame]
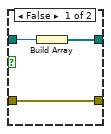
[diagram p5: hidden frame]
diagram:
  n1 = case shown="\"TDMS\"" "File Type" {
    tunnel: ["*.dat" ("pattern") "*.itx" ("pattern") "*.tdms" ("pattern") "*.vi" ("pattern")] -> w1
    frame "DAT", Default {
    }
    frame "ITX" {
    }
    frame "TDMS" {
    }
    frame "VI" {
    }
  }
  n2 = File/Directory Info(path="File or Folder Path") -> (directory=w5:bool, error out=w3:errorcluster)  [unwired: 1 in, 5 out]
  n3 = case shown="True" w5 {
    tunnel: [w14 w15] -> w6
    tunnel: "File or Folder Path" -> [w13 w19]
    tunnel: [w12 w18] -> w4
    tunnel: w3 -> [w12 w17]
    tunnel: w1 -> [_ w16]
    frame False {
      n4 = Build Array(w13) -> (w14:path[])
    }
    frame True {
      n5 = call <vilib>:"Recursive File List.vi"("pattern"=w16, "error in (no error)"=w17, "Folder Path"=w19) -> ("error out"=w18:errorcluster, "All Files in Dir"=w15:path[])  [unwired: 4 in, 3 out]
    }
  }
  n6 = while {
    tunnel: w6 -> [w63]
    tunnel: w4 -> [w58]
    stop <- "stop" stop-if-true
    # "Reverse array for interpolation to work for interpolation to work"
    n7 = Array Subset(array=w63, index="offset", length="length") -> (w59:path[])
    n8 = Array Size(array=w59) -> (size(s)=w62:i32)
    n9 = Divide(x=w62, y="decimate files") -> (x/y=w60:dbl)
    n10 = for {
      N: w60 -> [_]
      tunnel: w59 -> [w191]
      tunnel: [w191] -> _ mode=indexing
      tunnel: w58 -> [w186]
      tunnel: [w99] -> w54 mode=indexing
      tunnel: [w123] -> w48 mode=indexing
      tunnel: [w74] -> w21 mode=indexing
      tunnel: [w111] -> w56
      tunnel: [w100] -> w55 mode=indexing
      tunnel: [w98] -> w53 mode=indexing
      tunnel: [w97] -> w23 mode=indexing
      tunnel: [w96] -> w52 mode=indexing
      tunnel: [w95] -> w50 mode=indexing
      tunnel: [w94] -> w51 mode=indexing
      tunnel: [w93] -> w37 mode=indexing
      tunnel: [w88] -> w49 mode=indexing
      tunnel: [w85] -> w22 mode=indexing
      tunnel: [w78] -> w28
      tunnel: [w77] -> w24
      tunnel: [w76] -> w20 mode=indexing
      i -> [w188]
      w86 = TRUE ("averaging")
      w104 = 0 ("index")
      w126 = dbl[] []
      w172 = dbl[] []
      # "x axis"
      # "X axis graph"
      # "B"
      # "LG"
      # "BG"
      # "TG"
      n11 = local read "decimate files"() -> (w189:i32)
      n12 = Multiply(x=w189, y=w188) -> (x*y=w190:i32)
      n13 = Index Array(array=w191, index=w190) -> (element=w184:path)
      "Path" <- w184
      n14 = call <userlib>:"Data Read.vi"("Append Index"=-1, "error in (no error)"=w186, "path"=w184) -> ("error out"=w175:errorcluster, "Notes"=→"Comments":string, "Data (Dictionary)"=w183:T2[])  [unwired: 5 in, 1 out]
      "Data (Dictionary)" <- w183
      n15 = call <userlib>:"Dictionary Create__ogtk.vi"("error in (no error)"=w175, "initial dictionary (empty)"=w183) -> ("error out"=w132:errorcluster, "dictionary out"=w135:T5)  [unwired: 8 in]
      n16 = Unbundle By Name("index") -> ("Top gate"=w152:string, "Bottom Gate"=w151:string, "Local Gate"=w150:string, "B/Time"=w149:string, "X axis"=w144:string, "Temp"=w114:string)
      n17 = Unbundle By Name("index") -> ("I-(A)"=w171:string, "V4T-"=w170:string, "V4T+"=w169:string)
      n18 = call <userlib>:"Dictionary Get Value__ogtk.vi"("error in"=w132, "key"=w171, "dictionary"=w135) -> ("error out"=w178:errorcluster, "value"=w177:variant, "dictionary out"=w176:T5)  [unwired: 5 in, 1 out]
      n19 = Variant To Data(error in=w178, type=w172, Variant=w177) -> (data=w118:dbl[], error out=w174:errorcluster)
      n20 = call <userlib>:"Dictionary Get Value__ogtk.vi"("error in"=w174, "key"=w170, "dictionary"=w176) -> ("error out"=w182:errorcluster, "value"=w181:variant, "dictionary out"=w140:T5)  [unwired: 5 in, 1 out]
      n21 = Variant To Data(error in=w182, type=w172, Variant=w181) -> (data=w120:dbl[], error out=w173:errorcluster)
      n22 = call <userlib>:"Dictionary Get Value__ogtk.vi"("error in"=w173, "key"=w169, "dictionary"=w140) -> ("error out"=w180:errorcluster, "value"=w179:variant, "dictionary out"=w133:T5)  [unwired: 5 in, 1 out]
      n23 = call <userlib>:"Dictionary Get Value__ogtk.vi"("error in"=w132, "key"=w152, "dictionary"=w133) -> ("error out"=w156:errorcluster, "value"=w166:variant, "dictionary out"=w159:T5)  [unwired: 5 in, 1 out]
      n24 = Variant To Data(error in=w156, type=w126, Variant=w166) -> (data=w143:dbl[], error out=w155:errorcluster)
      n25 = call <userlib>:"Dictionary Get Value__ogtk.vi"("error in"=w155, "key"=w151, "dictionary"=w159) -> ("error out"=w161:errorcluster, "value"=w160:variant, "dictionary out"=w158:T5)  [unwired: 5 in, 1 out]
      n26 = Variant To Data(error in=w161, type=w126, Variant=w160) -> (data=w142:dbl[], error out=w154:errorcluster)
      n27 = call <userlib>:"Dictionary Get Value__ogtk.vi"("error in"=w154, "key"=w150, "dictionary"=w158) -> ("error out"=w165:errorcluster, "value"=w164:variant, "dictionary out"=w157:T5)  [unwired: 5 in, 1 out]
      n28 = Variant To Data(error in=w180, type=w172, Variant=w179) -> (data=w121:dbl[], error out=w78:errorcluster)
      n29 = Variant To Data(error in=w165, type=w126, Variant=w164) -> (data=w134:dbl[], error out=w153:errorcluster)
      n30 = call <userlib>:"Dictionary Get Value__ogtk.vi"("error in"=w153, "key"=w149, "dictionary"=w157) -> ("error out"=w163:errorcluster, "value"=w162:variant, "dictionary out"=w146:T5)  [unwired: 5 in, 1 out]
      n31 = Array Subset(array=w120, index="index", length="length") -> (w119:dbl[])
      n32 = Array Subset(array=w121, index="index", length="length") -> (w90:dbl[])
      n33 = Array Subset(array=w118, index="index", length="length") -> (w89:dbl[])
      n34 = Variant To Data(error in=w163, type=w126, Variant=w162) -> (data=w105:dbl[], error out=w145:errorcluster)
      n35 = Subtract(x=w90, y=w119) -> (x-y=w168:dbl[])
      n36 = Divide(x=w90, y=w89) -> (x/y=w87:dbl[])
      n37 = call <userlib>:"Dictionary Get Value__ogtk.vi"("error in"=w145, "key"=w144, "dictionary"=w146) -> ("error out"=w147:errorcluster, "value"=w148:variant, "dictionary out"=w130:T5)  [unwired: 5 in, 1 out]
      n38 = Select(t=w168, s="SE?", f=w90) -> (s? t:f=w103:dbl[])
      n39 = Variant To Data(error in=w147, type=w126, Variant=w148) -> (data=w77:dbl[], error out=w125:errorcluster)
      n40 = Array Subset(array=w77, index="index", length="length") -> (w102:dbl[])
      n41 = call-poly <vilib>:"Decimate (single shot).vi"("averaging"=w86, "decimating factor"="decimating factor", "X"=w102) -> ("Decimated Array"=w75:dbl[])  [unwired: 7 in, 1 out]
      n42 = call-poly <vilib>:"Decimate (single shot).vi"("averaging"=w86, "decimating factor"="decimating factor", "X"=w89) -> ("Decimated Array"=w83:dbl[])  [unwired: 7 in, 1 out]
      n43 = call-poly <vilib>:"Decimate (single shot).vi"("averaging"=w86, "decimating factor"="decimating factor", "X"=w103) -> ("Decimated Array"=w80:dbl[])  [unwired: 7 in, 1 out]
      n44 = Index Array(array=w143, index=w104) -> (element=w139:dbl)
      n45 = Index Array(array=w142, index=w104) -> (element=w137:dbl)
      n46 = Index Array(array=w134, index=w104) -> (element=w138:dbl)
      n47 = Index Array(array=w105, index=w104) -> (element=w136:dbl)
      n48 = Index Array(array=w77, index=w104) -> (element=w131:dbl)
      n49 = call <userlib>:"Dictionary Get Value__ogtk.vi"("error in"=w125, "key"=w114, "dictionary"=w130) -> ("error out"=w124:errorcluster, "value"=w127:variant, "dictionary out"=w129:T5)  [unwired: 5 in, 1 out]
      n50 = case shown="True" "Invert the voltage?" {
        tunnel: w80 -> [w192 w193]
        tunnel: [w192 w194] -> w79
        frame False {
        }
        frame True {
          n51 = Negate(x=w193) -> (-x=w194:dbl[])
        }
      }
      n52 = Divide(x=w83, y=w79) -> (x/y=w122:dbl[])
      n53 = Multiply(x=1.0, y=w122) -> (x*y=w108:dbl[])
      n54 = Bundle("Decimated Array"=w75, w87) -> (w88:cluster{"Decimated Array":dbl[], dbl[]})  [unwired: 1 in]
      n55 = Variant To Data(error in=w124, type=w126, Variant=w127) -> (data=w113:dbl[], error out=w115:errorcluster)
      n56 = Bundle("Decimated Array"=w75, w108) -> (w99:cluster{"Decimated Array":dbl[], dbl[]})  [unwired: 1 in]
      n57 = Reciprocal(x=w122) -> (1/x=w91:dbl[])
      n58 = Bundle("Decimated Array"=w75, "Decimated Array"=w83) -> (w123:T6)  [unwired: 1 in]
      n59 = Bundle("Decimated Array"=w75, "Decimated Array"=w79) -> (w74:T6)  [unwired: 1 in]
      n60 = disable-structure shown="Enabled" {
        disable-tunnel: [w206 _] -> w98
        disable-tunnel: [w205 _] -> w97
        disable-tunnel: [w204 _] -> w96
        disable-tunnel: [w202 _] -> w95
        disable-tunnel: [w197 _] -> w94
        disable-tunnel: [w195 _] -> _
        disable-tunnel: w74 -> [w195 _]
        frame Enabled {
          # "hhkk"
          n61 = call <userlib>:"Sort (single).vi"("XY-data"=w195) -> ("Sorted XY-data out"=w196:cluster{"X-array":dbl[], "Y-array":dbl[]})  [unwired: 8 in, 2 out]
          n62 = call "Symmetrize (multiple)_aditi.vi"("XY-data"=w196) -> ("Antisymmetric"=w205:cluster{"X-array":dbl[], "Y-array":dbl[]}, "Symmetric"=w206:cluster{"X-array":dbl[], "Y-array":dbl[]}, "XY-data out"=w197:cluster{"X-array":dbl[], "Y-array":dbl[]})  [unwired: 7 in, 1 out]
          n63 = Unbundle By Name(w206) -> ("X-array"=w201:dbl[], "Y-array"=w199:dbl[])
          n64 = Unbundle By Name(w205) -> ("Y-array"=w198:dbl[])
          n65 = Subtract(x=w199, y=w198) -> (x-y=w200:dbl[])
          n66 = Add(x=w199, y=w198) -> (x+y=w203:dbl[])
          n67 = Bundle("X-array"=w201, w200) -> (w202:cluster{"X-array":dbl[], dbl[]})  [unwired: 1 in]
          n68 = Bundle("X-array"=w201, w203) -> (w204:cluster{"X-array":dbl[], dbl[]})  [unwired: 1 in]
        }
        frame Disabled {
          # "Enable if you want Rsym Rantisym"
        }
      }
      n69 = local read "index"() -> (w110:i32)
      n70 = local read "length"() -> (w109:i32)
      n71 = Bundle("Decimated Array"=w75, w91) -> (w76:cluster{"Decimated Array":dbl[], dbl[]})  [unwired: 1 in]
      n72 = Array Subset(array=w113, index=w110, length=w109) -> (w112:dbl[])
      n73 = call <userlib>:"Dictionary Destroy__ogtk.vi"("error in (no error)"=w115, "dictionary"=w129) -> ()  [unwired: 9 in, 1 out]
      n74 = Reciprocal(x=w75) -> (1/x=w92:dbl[])
      n75 = Divide(x="Vac source", y=w83) -> (x/y=w82:dbl[])
      n76 = Array Subset(array=w105) -> (w106:dbl[])  [unwired: 2 in]
      n77 = Bundle(w92, w91) -> (w93:cluster{dbl[], dbl[]})  [unwired: 1 in]
      n78 = Bundle("Decimated Array"=w79, "Decimated Array"=w83) -> (w100:T6)  [unwired: 1 in]
      n79 = Bundle(w139, w137, w138, w136, w131) -> (→"Gates and B":cluster{dbl, dbl, dbl, dbl, dbl})  [unwired: 1 in]
      n80 = Bundle("Decimated Array"=w75, w82) -> (w85:cluster{"Decimated Array":dbl[], dbl[]})  [unwired: 1 in]
      n81 = Bundle(w106, w112) -> (w111:cluster{dbl[], dbl[]})  [unwired: 1 in]
      "counter" <- w188
    }
    "V_N vs B" <- w21
    "Gvs B" <- w54
    "Temp vs Field/Time" <- w56
    "I vs  B" <- w48
    "I V4" <- w55
    "R vs B Anti" <- w23
    "R vs Bsym" <- w53
    "Sum" <- w52
    "Diff" <- w50
    "R vs B out" <- w51
    "R vs 1/B" <- w37
    "V/I vs Vsg" <- w49
    "R4T" <- w20
    "R2T vs T" <- w22
    n82 = disable-structure shown="Disabled" {
      disable-tunnel: w37 -> [w73 _]
      frame Disabled {
        (unwired) TRUE ("restart averaging (F)")
        n83 = Index Array(array=w73) -> (element=w68:cluster{dbl[], dbl[]})  [unwired: 1 in]
        n84 = call-poly <userlib>:"Sort.vi"("XY-data"=w68) -> ("Sorted XY-data out"=w72:cluster{"X-array":dbl[], "Y-array":dbl[]})  [unwired: 8 in, 2 out]
        n85 = call <userlib>:"Resample (single).vi"("t0"=-3.32, "dt"=0.01, "XY-data"=w72) -> ("error out"=w70:errorcluster, "Resampled XY-data out"=w71:cluster{"X-array":dbl[], "Y-array":dbl[]})  [unwired: 7 in]
        "R vs 1/B 2" <- w71
        n86 = call <userlib>:"FFT (single).vi"("error in (no error)"=w70, "XY-data"=w71) -> ("magnitude"=→"Waveform Graph 2":cluster{"f0":dbl, "df":dbl, "magnitude":dbl[]})  [unwired: 6 in, 3 out]
      }
      frame Enabled {
      }
    }
    n87 = call-poly <userlib>:"Sort.vi"("error in (no error)"=w28, "XY-data"=w21) -> ("error out"=w29:errorcluster, "Sorted XY-data out"=w27:cluster{"X-array":dbl[], "Y-array":dbl[]}[])  [unwired: 7 in, 1 out]
    n88 = call-poly <userlib>:"Sort.vi"("error in (no error)"=w28, "XY-data"=w20) -> ("error out"=w30:errorcluster, "Sorted XY-data out"=w31:cluster{"X-array":dbl[], "Y-array":dbl[]}[])  [unwired: 7 in, 1 out]
    n89 = call-poly <userlib>:"Moving Average.vi"("error in (no error)"=w29, "Window"="Averaging", "XY-data"=w27) -> ("error out"=w34:errorcluster, "XY-data out"=w44:cluster{"X-array":dbl[], "Y-array":dbl[]}[])  [unwired: 7 in]
    n90 = control-ref of="Nernst"() -> (w32:refnum<vi>)
    n91 = control-ref of="R4T"() -> (w38:refnum<vi>)
    n92 = call <userlib>:"XY to 2D.vi"("error in (no error)"=w30, "Fake Point"=0.0, "Interpolate [T]"="Interpolate [T]", "XY-data"=w31) -> ("error out"=w39:errorcluster, "2D Y Array"=→"R4T":dbl[][])  [unwired: 4 in, 2 out]
    n93 = call <userlib>:"XY to 2D.vi"("error in (no error)"=w34, "Fake Point"=0.0, "Interpolate [T]"="Interpolate [T]", "XY-data"=w44) -> ("error out"=w33:errorcluster, "2D Y Array"=→"Nernst":dbl[][])  [unwired: 4 in, 2 out]
    n94 = call <userlib>:"Write Intensity Graph ref.vi"("error in (no error)"=w39, "Intensity Graph"=w38) -> ("error out"=w40:errorcluster, "graph_utilities out"=w41:refnum<class "graph_utilities.lvclass">)  [unwired: 8 in]
    n95 = Sort 1D Array(array=w24) -> (sorted array=w25:dbl[])
    n96 = call <userlib>:"Write Intensity Graph ref.vi"("error in (no error)"=w33, "Intensity Graph"=w32) -> ("error out"=w35:errorcluster, "graph_utilities out"=w36:refnum<class "graph_utilities.lvclass">)  [unwired: 8 in]
    n97 = call <userlib>:"Set Intensity Graph X Scale Array.vi"("error in (no error)"=w40, "X Scale"=w25, "graph_utilities in"=w41) -> ()  [unwired: 7 in, 2 out]
    n98 = call <userlib>:"Set Intensity Graph X Scale Array.vi"("error in (no error)"=w35, "X Scale"=w25, "graph_utilities in"=w36) -> ()  [unwired: 7 in, 2 out]
  }
